vi "app - Scott Thing.vi"() -> ()   [LabVIEW 2014]
uses:
  <vilib>/event_ctls.llb/eventvkey.ctl
  freq file -- file select control.ctl
  freq file -- file select folder control.ctl
  cursor winow.ctl
  fit function selector control.ctl
  countdown control.ctl
  cursor window action.ctl
  array transformation action.ctl
  container action.ctl
  cursor action.ctl
  save-read action.ctl
  generate linear region.vi
  tale of three indices.vi
  Q -- check range -- i -- real.vi
  linear interpolation iiii- complex.vi
  Q -- check range -- i -- integer.vi
  file -- 9w path.vi
  file -- open-create folder.vi
  command stack.vi
  tale of three indices -- check state.vi
  Q - not nan -- real.vi
  Q - not nan -- integer.vi
  <vilib>/regexp/Match Regular Expression.xnode
panel:
  in  "plot fit?":bool
  out "slope temp vs time (K/min)":dbl=-0.40469687981224706
  out "slope vs temp (1/K)":dbl=-8.892288495374525e-05
  out "slope vs time (1/min)":dbl=3.599048348461236e-05
  in  "phase":dbl=10.0
  out "phase of Frequency vs Temperature phase(rad)":dbl=10.0
  out "phase of Frequency (rad)":dbl=10.0
  out "phase of Temperature (rad)":dbl=10.0
  in  "window/period":dbl=114.59
  out "averaging window (min)":dbl=114.59
  in  "cursor bracket: delta freq vs time":T1={"left"=45.0, "right "=55.0, "center"=50.0, "window"=10.0, "cursors"=[1, 2, 3], "relative"=0, "absolute"=0, "fixed vertical offset"=0.0, "vertical offset"=0.0, "skew"=0.0, "default window frac"=0.1, "kind"=enum."skewed", "skew.left"=0.5, "skew.right"=0.5, "Plot ref"=refnum, "wing order"=enum."forw"}
  in  "period (min)":dbl(slide) scale=0.0..200.0
  in  "Lockin wave: Period (min)":dbl=114.59
  in  "Lockin wave: Amplitude":dbl=10.0
  in  "Lockin wave: Phase":dbl=1.0
  in  "lockin (l)":bool
  out "Plot: lockin":cluster{dbl[], dbl[]}[](graph)
  in  "Numeric sort  folder names ?":bool=TRUE
  in  "Tab : other":enum32{"indicators", "other"}(tab)
  in  "file 2 (red)":T2={"from file "="890_mo", "load"=TRUE, "read from file list"=3, "folder kind"=enum."monitor"} {"read from file list" items=["363_mo", "524_mo", "997_mo", "1331_mo", "2102_mo", "2312_mo", "3182_mo", "3227_mo", "3271_mo", "3302_mo", "3420_mo", "3606_mo", "3780_mo", "3988_mo"]}
  in  "file 1 (blue)":T2={"from file "="890_mo", "load"=TRUE, "read from file list"=3, "folder kind"=enum."monitor"} {"read from file list" items=["363_mo", "524_mo", "997_mo", "1331_mo", "2102_mo", "2312_mo", "3182_mo", "3227_mo", "3271_mo", "3302_mo", "3420_mo", "3606_mo", "3780_mo", "3988_mo"]}
  out "time (min)":dbl=513.2382892057026
  in  "open (o)":bool
  in  "plot (p)":bool
  in  "plot type":T4(ring)=enum."plot vs Temperature"
  out "temperature (K)":dbl=369.642
  out "frequency (kHz)":dbl
  in  "sweep folder 2":u16(ring)=1 items=["0_test", "1_cooling", "2_heating", "3_heating"]
  in  "sweep folder 1":u16(ring)=1 items=["0_test", "1_cooling", "2_heating", "3_heating"]
  out "folder --OK":bool=TRUE
  out "file 2 -- OK":bool=TRUE
  out "file 1 -- OK":bool=TRUE
  out "best fit parameters":dbl[](array[numeric])=[61.921916709262796, 419.38173960994607, 184.61021915940464]
  in  "fit dataset":enum16{"fit blue dataset", "fit red  dataset"}(ring)
  in  "fit using":T5=enum."einstein"
  out "current index":dbl=1431.5698546544484
  out "Char":i16=122
  out "VKey":T6
  in  "Tab: timer":enum32{"timer ON", "timer OFF"}(tab)=enum."timer OFF"
  in  "timer  \"update\"":dbl(slide) min=-543877211.0 max=2129711151.0 step=0.010000000000000002 scale=0.0..100.0 scale format="%#3_3f"
  in  "Tab : all":enum32{"everything", "everything else"}(tab)
  out "Plot: gamma vs time":cluster{dbl[], dbl[]}[](graph)=[{[0.0, 0.8321000039577484, 1.8338100016117096, 2.665260002017021, 3.6651000007987022, 4.500330001115799, 5.331799998879433, 6.33356000483036, 7.165059998631477, 8.166830003261566, 9.000310003757477, 9.665630005300045, 10.330900005996227, 10.99813000112772, 11.66363000124693, 12.332860000431538, 12.833530001342297, 13.498850002884865, 14.16593000292778, 14.831310003995895, 15.49855000525713, 16.165710002183914, 16.833000004291534, 17.33186000585556, 17.999030001461506, 18.66473000496626, 19.331909999251366, 19.99728000164032, 20.66636000573635, 21.33170000463724, 21.83238000422716, 22.49956000596285, 23.164850004017353, 23.83196000009775, 24.499110005795956, 25.16636000573635, 25.831660002470016, 26.332430005073547, 26.999680005013943, 27.664980001747608, 28.334049999713898, 28.99931000173092, 29.66651000082493, 30.331810005009174, 30.832600004971027, 31.49796000123024, 32.165130004286766, 32.83415000140667, 33.49946000427008, 34.166660003364086, 34.831980004906654, 35.332830004394054, 35.99830999970436, 36.667510002851486, 37.33306000381708, 38.000459998846054, 38.665800005197525, 39.33306000381708, 39.83373000472784, 40.499180004000664, 41.16650000214577, 41.83186000585556, 42.500900000333786, 43.166230000555515, 43.833429999649525, 44.332249999046326, 44.99943000078201, 45.66485000401735, 46.334100000560284, 46.99949999898672, 47.6666100025177, 47.982130005955696, 48.19973000138998, 48.33212999999523, 48.83280999958515, 49.50008000433445, 50.16723000258207, 50.834449999034405, 51.49991000443697, 52.16526000201702, 52.83435000479221, 53.33311000466347, 54.0003300011158, 54.66745000332594, 55.33465000241995, 55.999960005283356, 56.66730999946594, 57.33255000412464, 57.83314999938011, 58.50026000291109, 59.16743000596762, 59.83455999940634, 60.499880000948906, 61.16710000485182, 61.83251000195742, 62.33313000202179, 63.002580001950264, 63.667830005288124, 64.33306000381708, 65.00022999942303, 65.66740000247955, 66.33458000421524, 66.83331000059843, 67.50053000450134, 68.16818000376225, 68.83345000445843, 69.50058000534773, 70.16781000047922, 70.83495999872684, 71.33570000529289, 72.00148000568151, 72.66678000241518, 73.33390000462532, 74.00111000239849, 74.66830000281334, 75.33545999974012, 75.8344499990344, 76.50161000341177, 77.16766000539064, 77.83305000513792, 78.50201000273228, 79.1691600009799, 79.83455000072718, 80.33545999974012, 81.00163000077009, 81.66701000183821, 82.33430000394583, 83.00148000568151, 83.66863000392914, 84.33410999923944, 84.8347800001502, 85.50213000178337, 86.1676000058651, 86.83668000251055, 87.5020300000906, 88.16926000267267, 88.83460000157356, 89.33528000116348, 90.00060000270605, 90.66975000500679, 91.33512999862432, 92.00230000168085, 92.66781000047922, 93.33495999872684, 93.83557999879122, 94.50090999901295, 95.16995999962091, 95.83531000465155, 96.50246000289917, 97.16770000010729, 97.83486000448465, 98.33560000360012, 99.00268000364304, 99.66976000368595, 100.33528000116348, 101.06157000362873], [0.67588, 0.61324, 0.61184, 0.55194, 0.46793, 0.65413, 0.45513, 0.53529, 0.55031, 0.6231, 0.46874, 0.37253, 0.62303, 0.69213, 0.48939, 0.40586, 0.51301, 0.53019, 0.56055, 0.71323, 0.4387, 0.62201, 0.52499, 0.55885, 0.40767, 0.52913, 0.37684, 0.81007, 0.55143, 0.62952, 0.6183, 0.66198, 0.55623, 0.41442, 0.51737, 0.49906, 0.34582, 0.55383, 0.50878, 0.61849, 0.46781, 0.4094, 0.56226, 0.53343, 0.56808, 0.59375, 0.55552, 0.52806, 0.55238, 0.57542, 0.55055, 0.51811, 0.56627, 0.47603, 0.60558, 0.5391, 0.53997, 0.46766, 0.50061, 0.55367, 0.54193, 0.57806, 0.59611, 0.41969, 0.60712, 0.57486, 0.54068, 0.49673, 0.41822, 0.51666, 0.53002, 0.54071, 0.54381, 0.50371, 0.47659, 0.55271, 0.51695, 0.5054, 0.48403, 0.63454, 0.46381, 0.54415, 0.49407, 0.50294, 0.59277, 0.51141, 0.49779, 0.62513, 0.58238, 0.60458, 0.51762, 0.49132, 0.62927, 0.59156, 0.61264, 0.58665, 0.49186, 0.57277, 0.60236, 0.52088, 0.54777, 0.34446, 0.60604, 0.56549, 0.5463, 0.62015, 0.55365, 0.55892, 0.59896, 0.5722, 0.6325, 0.52149, 0.60349, 0.49569, 0.5793, 0.6434, 0.58917, 0.56576, 0.62655, 0.66023, 0.6492, 0.64793, 0.66476, 0.61207, 0.69632, 0.68932, 0.6121, 0.67902, 0.6855, 0.6683, 0.68361, 0.71016, 0.731, 0.74257, 0.71351, 0.66404, 0.77828, 0.66741, 0.65821, 0.79074, 0.71129, 0.70388, 0.704, 0.73193, 0.7246, 0.75975, 0.76321, 0.75811, 0.69136, 0.71185, 0.76071, 0.59918, 0.80205, 0.73634, 0.77823, 0.66937]}]
  out "Plot: temp vs time":cluster{dbl[], dbl[]}[](graph)=[{[0.0, 0.8321000039577484, 1.8338100016117096, 2.665260002017021, 3.6651000007987022, 4.500330001115799, 5.331799998879433, 6.33356000483036, 7.165059998631477, 8.166830003261566, 9.000310003757477, 9.665630005300045, 10.330900005996227, 10.99813000112772, 11.66363000124693, 12.332860000431538, 12.833530001342297, 13.498850002884865, 14.16593000292778, 14.831310003995895, 15.49855000525713, 16.165710002183914, 16.833000004291534, 17.33186000585556, 17.999030001461506, 18.66473000496626, 19.331909999251366, 19.99728000164032, 20.66636000573635, 21.33170000463724, 21.83238000422716, 22.49956000596285, 23.164850004017353, 23.83196000009775, 24.499110005795956, 25.16636000573635, 25.831660002470016, 26.332430005073547, 26.999680005013943, 27.664980001747608, 28.334049999713898, 28.99931000173092, 29.66651000082493, 30.331810005009174, 30.832600004971027, 31.49796000123024, 32.165130004286766, 32.83415000140667, 33.49946000427008, 34.166660003364086, 34.831980004906654, 35.332830004394054, 35.99830999970436, 36.667510002851486, 37.33306000381708, 38.000459998846054, 38.665800005197525, 39.33306000381708, 39.83373000472784, 40.499180004000664, 41.16650000214577, 41.83186000585556, 42.500900000333786, 43.166230000555515, 43.833429999649525, 44.332249999046326, 44.99943000078201, 45.66485000401735, 46.334100000560284, 46.99949999898672, 47.6666100025177, 47.982130005955696, 48.19973000138998, 48.33212999999523, 48.83280999958515, 49.50008000433445, 50.16723000258207, 50.834449999034405, 51.49991000443697, 52.16526000201702, 52.83435000479221, 53.33311000466347, 54.0003300011158, 54.66745000332594, 55.33465000241995, 55.999960005283356, 56.66730999946594, 57.33255000412464, 57.83314999938011, 58.50026000291109, 59.16743000596762, 59.83455999940634, 60.499880000948906, 61.16710000485182, 61.83251000195742, 62.33313000202179, 63.002580001950264, 63.667830005288124, 64.33306000381708, 65.00022999942303, 65.66740000247955, 66.33458000421524, 66.83331000059843, 67.50053000450134, 68.16818000376225, 68.83345000445843, 69.50058000534773, 70.16781000047922, 70.83495999872684, 71.33570000529289, 72.00148000568151, 72.66678000241518, 73.33390000462532, 74.00111000239849, 74.66830000281334, 75.33545999974012, 75.8344499990344, 76.50161000341177, 77.16766000539064, 77.83305000513792, 78.50201000273228, 79.1691600009799, 79.83455000072718, 80.33545999974012, 81.00163000077009, 81.66701000183821, 82.33430000394583, 83.00148000568151, 83.66863000392914, 84.33410999923944, 84.8347800001502, 85.50213000178337, 86.1676000058651, 86.83668000251055, 87.5020300000906, 88.16926000267267, 88.83460000157356, 89.33528000116348, 90.00060000270605, 90.66975000500679, 91.33512999862432, 92.00230000168085, 92.66781000047922, 93.33495999872684, 93.83557999879122, 94.50090999901295, 95.16995999962091, 95.83531000465155, 96.50246000289917, 97.16770000010729, 97.83486000448465, 98.33560000360012, 99.00268000364304, 99.66976000368595, 100.33528000116348, 101.06157000362873], [306.859, 306.865, 306.758, 306.535, 306.258, 305.982, 305.68, 305.339, 305.019, 304.645, 304.3, 303.965, 303.725, 303.462, 303.2, 302.977, 302.732, 302.46, 302.218, 301.952, 301.736, 301.437, 301.186, 300.927, 300.684, 300.432, 300.14, 299.908, 299.659, 299.377, 299.116, 298.866, 298.605, 298.361, 298.06, 297.801, 297.575, 297.284, 297.046, 296.769, 296.514, 296.224, 295.989, 295.704, 295.444, 295.182, 294.904, 294.655, 294.379, 294.131, 293.821, 293.569, 293.289, 293.052, 292.75, 292.472, 292.244, 291.771, 291.552, 291.447, 291.24, 290.887, 290.534, 290.294, 290.021, 289.766, 289.473, 289.178, 288.91, 288.631, 288.354, 288.354, 288.354, 288.104, 287.889, 287.626, 287.379, 287.122, 286.875, 286.621, 286.387, 286.134, 285.896, 285.647, 285.385, 285.15, 284.882, 284.657, 284.389, 284.134, 283.88, 283.628, 283.367, 283.103, 282.849, 282.604, 282.322, 282.068, 281.815, 281.535, 281.296, 281.007, 280.774, 280.511, 280.222, 279.971, 279.687, 279.464, 279.175, 278.934, 278.648, 278.394, 278.136, 277.881, 277.611, 277.368, 277.093, 276.842, 276.498, 276.243, 276.006, 275.757, 275.403, 275.18, 274.898, 274.596, 274.32, 274.065, 273.786, 273.463, 273.219, 272.879, 272.671, 272.345, 272.085, 271.771, 271.544, 271.227, 270.941, 270.676, 270.353, 270.079, 269.753, 269.519, 269.228, 268.904, 268.594, 268.306, 268.058, 267.801, 267.52, 267.286, 267.028, 266.779, 266.494, 266.257]}]
  out "Plot: gamma":cluster{dbl[], dbl[]}[](graph)=[{[306.859, 306.865, 306.758, 306.535, 306.258, 305.982, 305.68, 305.339, 305.019, 304.645, 304.3, 303.965, 303.725, 303.462, 303.2, 302.977, 302.732, 302.46, 302.218, 301.952, 301.736, 301.437, 301.186, 300.927, 300.684, 300.432, 300.14, 299.908, 299.659, 299.377, 299.116, 298.866, 298.605, 298.361, 298.06, 297.801, 297.575, 297.284, 297.046, 296.769, 296.514, 296.224, 295.989, 295.704, 295.444, 295.182, 294.904, 294.655, 294.379, 294.131, 293.821, 293.569, 293.289, 293.052, 292.75, 292.472, 292.244, 291.771, 291.552, 291.447, 291.24, 290.887, 290.534, 290.294, 290.021, 289.766, 289.473, 289.178, 288.91, 288.631, 288.354, 288.354, 288.354, 288.104, 287.889, 287.626, 287.379, 287.122, 286.875, 286.621, 286.387, 286.134, 285.896, 285.647, 285.385, 285.15, 284.882, 284.657, 284.389, 284.134, 283.88, 283.628, 283.367, 283.103, 282.849, 282.604, 282.322, 282.068, 281.815, 281.535, 281.296, 281.007, 280.774, 280.511, 280.222, 279.971, 279.687, 279.464, 279.175, 278.934, 278.648, 278.394, 278.136, 277.881, 277.611, 277.368, 277.093, 276.842, 276.498, 276.243, 276.006, 275.757, 275.403, 275.18, 274.898, 274.596, 274.32, 274.065, 273.786, 273.463, 273.219, 272.879, 272.671, 272.345, 272.085, 271.771, 271.544, 271.227, 270.941, 270.676, 270.353, 270.079, 269.753, 269.519, 269.228, 268.904, 268.594, 268.306, 268.058, 267.801, 267.52, 267.286, 267.028, 266.779, 266.494, 266.257], [0.67588, 0.61324, 0.61184, 0.55194, 0.46793, 0.65413, 0.45513, 0.53529, 0.55031, 0.6231, 0.46874, 0.37253, 0.62303, 0.69213, 0.48939, 0.40586, 0.51301, 0.53019, 0.56055, 0.71323, 0.4387, 0.62201, 0.52499, 0.55885, 0.40767, 0.52913, 0.37684, 0.81007, 0.55143, 0.62952, 0.6183, 0.66198, 0.55623, 0.41442, 0.51737, 0.49906, 0.34582, 0.55383, 0.50878, 0.61849, 0.46781, 0.4094, 0.56226, 0.53343, 0.56808, 0.59375, 0.55552, 0.52806, 0.55238, 0.57542, 0.55055, 0.51811, 0.56627, 0.47603, 0.60558, 0.5391, 0.53997, 0.46766, 0.50061, 0.55367, 0.54193, 0.57806, 0.59611, 0.41969, 0.60712, 0.57486, 0.54068, 0.49673, 0.41822, 0.51666, 0.53002, 0.54071, 0.54381, 0.50371, 0.47659, 0.55271, 0.51695, 0.5054, 0.48403, 0.63454, 0.46381, 0.54415, 0.49407, 0.50294, 0.59277, 0.51141, 0.49779, 0.62513, 0.58238, 0.60458, 0.51762, 0.49132, 0.62927, 0.59156, 0.61264, 0.58665, 0.49186, 0.57277, 0.60236, 0.52088, 0.54777, 0.34446, 0.60604, 0.56549, 0.5463, 0.62015, 0.55365, 0.55892, 0.59896, 0.5722, 0.6325, 0.52149, 0.60349, 0.49569, 0.5793, 0.6434, 0.58917, 0.56576, 0.62655, 0.66023, 0.6492, 0.64793, 0.66476, 0.61207, 0.69632, 0.68932, 0.6121, 0.67902, 0.6855, 0.6683, 0.68361, 0.71016, 0.731, 0.74257, 0.71351, 0.66404, 0.77828, 0.66741, 0.65821, 0.79074, 0.71129, 0.70388, 0.704, 0.73193, 0.7246, 0.75975, 0.76321, 0.75811, 0.69136, 0.71185, 0.76071, 0.59918, 0.80205, 0.73634, 0.77823, 0.66937]}, {[306.859, 306.865, 306.758, 306.535, 306.258, 305.982, 305.68, 305.339, 305.019, 304.645, 304.3, 303.965, 303.725, 303.462, 303.2, 302.977, 302.732, 302.46, 302.218, 301.952, 301.736, 301.437, 301.186, 300.927, 300.684, 300.432, 300.14, 299.908, 299.659, 299.377, 299.116, 298.866, 298.605, 298.361, 298.06, 297.801, 297.575, 297.284, 297.046, 296.769, 296.514, 296.224, 295.989, 295.704, 295.444, 295.182, 294.904, 294.655, 294.379, 294.131, 293.821, 293.569, 293.289, 293.052, 292.75, 292.472, 292.244, 291.771, 291.552, 291.447, 291.24, 290.887, 290.534, 290.294, 290.021, 289.766, 289.473, 289.178, 288.91, 288.631, 288.354, 288.354, 288.354, 288.104, 287.889, 287.626, 287.379, 287.122, 286.875, 286.621, 286.387, 286.134, 285.896, 285.647, 285.385, 285.15, 284.882, 284.657, 284.389, 284.134, 283.88, 283.628, 283.367, 283.103, 282.849, 282.604, 282.322, 282.068, 281.815, 281.535, 281.296, 281.007, 280.774, 280.511, 280.222, 279.971, 279.687, 279.464, 279.175, 278.934, 278.648, 278.394, 278.136, 277.881, 277.611, 277.368, 277.093, 276.842, 276.498, 276.243, 276.006, 275.757, 275.403, 275.18, 274.898, 274.596, 274.32, 274.065, 273.786, 273.463, 273.219, 272.879, 272.671, 272.345, 272.085, 271.771, 271.544, 271.227, 270.941, 270.676, 270.353, 270.079, 269.753, 269.519, 269.228, 268.904, 268.594, 268.306, 268.058, 267.801, 267.52, 267.286, 267.028, 266.779, 266.494, 266.257], [0.67588, 0.61324, 0.61184, 0.55194, 0.46793, 0.65413, 0.45513, 0.53529, 0.55031, 0.6231, 0.46874, 0.37253, 0.62303, 0.69213, 0.48939, 0.40586, 0.51301, 0.53019, 0.56055, 0.71323, 0.4387, 0.62201, 0.52499, 0.55885, 0.40767, 0.52913, 0.37684, 0.81007, 0.55143, 0.62952, 0.6183, 0.66198, 0.55623, 0.41442, 0.51737, 0.49906, 0.34582, 0.55383, 0.50878, 0.61849, 0.46781, 0.4094, 0.56226, 0.53343, 0.56808, 0.59375, 0.55552, 0.52806, 0.55238, 0.57542, 0.55055, 0.51811, 0.56627, 0.47603, 0.60558, 0.5391, 0.53997, 0.46766, 0.50061, 0.55367, 0.54193, 0.57806, 0.59611, 0.41969, 0.60712, 0.57486, 0.54068, 0.49673, 0.41822, 0.51666, 0.53002, 0.54071, 0.54381, 0.50371, 0.47659, 0.55271, 0.51695, 0.5054, 0.48403, 0.63454, 0.46381, 0.54415, 0.49407, 0.50294, 0.59277, 0.51141, 0.49779, 0.62513, 0.58238, 0.60458, 0.51762, 0.49132, 0.62927, 0.59156, 0.61264, 0.58665, 0.49186, 0.57277, 0.60236, 0.52088, 0.54777, 0.34446, 0.60604, 0.56549, 0.5463, 0.62015, 0.55365, 0.55892, 0.59896, 0.5722, 0.6325, 0.52149, 0.60349, 0.49569, 0.5793, 0.6434, 0.58917, 0.56576, 0.62655, 0.66023, 0.6492, 0.64793, 0.66476, 0.61207, 0.69632, 0.68932, 0.6121, 0.67902, 0.6855, 0.6683, 0.68361, 0.71016, 0.731, 0.74257, 0.71351, 0.66404, 0.77828, 0.66741, 0.65821, 0.79074, 0.71129, 0.70388, 0.704, 0.73193, 0.7246, 0.75975, 0.76321, 0.75811, 0.69136, 0.71185, 0.76071, 0.59918, 0.80205, 0.73634, 0.77823, 0.66937]}]
  out "Plot: freq vs time":cluster{dbl[], dbl[]}[](graph)=[{[0.0, 0.8321000039577484, 1.8338100016117096, 2.665260002017021, 3.6651000007987022, 4.500330001115799, 5.331799998879433, 6.33356000483036, 7.165059998631477, 8.166830003261566, 9.000310003757477, 9.665630005300045, 10.330900005996227, 10.99813000112772, 11.66363000124693, 12.332860000431538, 12.833530001342297, 13.498850002884865, 14.16593000292778, 14.831310003995895, 15.49855000525713, 16.165710002183914, 16.833000004291534, 17.33186000585556, 17.999030001461506, 18.66473000496626, 19.331909999251366, 19.99728000164032, 20.66636000573635, 21.33170000463724, 21.83238000422716, 22.49956000596285, 23.164850004017353, 23.83196000009775, 24.499110005795956, 25.16636000573635, 25.831660002470016, 26.332430005073547, 26.999680005013943, 27.664980001747608, 28.334049999713898, 28.99931000173092, 29.66651000082493, 30.331810005009174, 30.832600004971027, 31.49796000123024, 32.165130004286766, 32.83415000140667, 33.49946000427008, 34.166660003364086, 34.831980004906654, 35.332830004394054, 35.99830999970436, 36.667510002851486, 37.33306000381708, 38.000459998846054, 38.665800005197525, 39.33306000381708, 39.83373000472784, 40.499180004000664, 41.16650000214577, 41.83186000585556, 42.500900000333786, 43.166230000555515, 43.833429999649525, 44.332249999046326, 44.99943000078201, 45.66485000401735, 46.334100000560284, 46.99949999898672, 47.6666100025177, 47.982130005955696, 48.19973000138998, 48.33212999999523, 48.83280999958515, 49.50008000433445, 50.16723000258207, 50.834449999034405, 51.49991000443697, 52.16526000201702, 52.83435000479221, 53.33311000466347, 54.0003300011158, 54.66745000332594, 55.33465000241995, 55.999960005283356, 56.66730999946594, 57.33255000412464, 57.83314999938011, 58.50026000291109, 59.16743000596762, 59.83455999940634, 60.499880000948906, 61.16710000485182, 61.83251000195742, 62.33313000202179, 63.002580001950264, 63.667830005288124, 64.33306000381708, 65.00022999942303, 65.66740000247955, 66.33458000421524, 66.83331000059843, 67.50053000450134, 68.16818000376225, 68.83345000445843, 69.50058000534773, 70.16781000047922, 70.83495999872684, 71.33570000529289, 72.00148000568151, 72.66678000241518, 73.33390000462532, 74.00111000239849, 74.66830000281334, 75.33545999974012, 75.8344499990344, 76.50161000341177, 77.16766000539064, 77.83305000513792, 78.50201000273228, 79.1691600009799, 79.83455000072718, 80.33545999974012, 81.00163000077009, 81.66701000183821, 82.33430000394583, 83.00148000568151, 83.66863000392914, 84.33410999923944, 84.8347800001502, 85.50213000178337, 86.1676000058651, 86.83668000251055, 87.5020300000906, 88.16926000267267, 88.83460000157356, 89.33528000116348, 90.00060000270605, 90.66975000500679, 91.33512999862432, 92.00230000168085, 92.66781000047922, 93.33495999872684, 93.83557999879122, 94.50090999901295, 95.16995999962091, 95.83531000465155, 96.50246000289917, 97.16770000010729, 97.83486000448465, 98.33560000360012, 99.00268000364304, 99.66976000368595, 100.33528000116348, 101.06157000362873], [889.69584, 889.68006, 889.69255, 889.71739, 889.74198, 889.76413, 889.80509, 889.81267, 889.81316, 889.83768, 889.86543, 889.88159, 889.92939, 889.90105, 889.9266, 889.95895, 889.97981, 889.97629, 889.98977, 890.00084, 890.03646, 890.03085, 890.07055, 890.08625, 890.08815, 890.10584, 890.1305, 890.12034, 890.16981, 890.17806, 890.23087, 890.20536, 890.20895, 890.26922, 890.27026, 890.2972, 890.29936, 890.33499, 890.34497, 890.35023, 890.38545, 890.40235, 890.4306, 890.43746, 890.47621, 890.46739, 890.48511, 890.50908, 890.54654, 890.5436, 890.5795, 890.5927, 890.60709, 890.62748, 890.63996, 890.66299, 890.6957, 890.71803, 890.72686, 890.73173, 890.77668, 890.76873, 890.81256, 890.82914, 890.85272, 890.85398, 890.87546, 890.9031, 890.91221, 890.94167, 890.96276, 890.9639, 890.96372, 890.98604, 891.01233, 891.02469, 891.04793, 891.07006, 891.08048, 891.09899, 891.12512, 891.12536, 891.15654, 891.16879, 891.18905, 891.19959, 891.22995, 891.24753, 891.26162, 891.28335, 891.28567, 891.31231, 891.32899, 891.34942, 891.36424, 891.3683, 891.38547, 891.40448, 891.44656, 891.44488, 891.47205, 891.20744, 891.49222, 891.54408, 891.54113, 891.572, 891.58143, 891.60752, 891.60686, 891.64483, 891.65678, 891.68328, 891.6931, 891.70715, 891.72898, 891.75723, 891.77658, 891.78596, 891.81354, 891.83601, 891.85493, 891.86836, 891.88286, 891.89968, 891.93208, 891.95223, 891.96891, 891.99329, 892.01204, 892.02476, 892.05135, 892.06661, 892.06875, 892.09013, 892.12382, 892.14219, 892.1629, 892.18968, 892.20319, 892.24544, 892.25704, 892.28489, 892.29651, 892.31599, 892.33983, 892.34947, 892.37436, 892.40785, 892.42946, 892.4521, 892.46919, 892.48367, 892.49371, 892.51877, 892.53774, 892.56817]}]
  out "Plot: frequency":cluster{dbl[], dbl[]}[](graph)=[{[306.859, 306.865, 306.758, 306.535, 306.258, 305.982, 305.68, 305.339, 305.019, 304.645, 304.3, 303.965, 303.725, 303.462, 303.2, 302.977, 302.732, 302.46, 302.218, 301.952, 301.736, 301.437, 301.186, 300.927, 300.684, 300.432, 300.14, 299.908, 299.659, 299.377, 299.116, 298.866, 298.605, 298.361, 298.06, 297.801, 297.575, 297.284, 297.046, 296.769, 296.514, 296.224, 295.989, 295.704, 295.444, 295.182, 294.904, 294.655, 294.379, 294.131, 293.821, 293.569, 293.289, 293.052, 292.75, 292.472, 292.244, 291.771, 291.552, 291.447, 291.24, 290.887, 290.534, 290.294, 290.021, 289.766, 289.473, 289.178, 288.91, 288.631, 288.354, 288.354, 288.354, 288.104, 287.889, 287.626, 287.379, 287.122, 286.875, 286.621, 286.387, 286.134, 285.896, 285.647, 285.385, 285.15, 284.882, 284.657, 284.389, 284.134, 283.88, 283.628, 283.367, 283.103, 282.849, 282.604, 282.322, 282.068, 281.815, 281.535, 281.296, 281.007, 280.774, 280.511, 280.222, 279.971, 279.687, 279.464, 279.175, 278.934, 278.648, 278.394, 278.136, 277.881, 277.611, 277.368, 277.093, 276.842, 276.498, 276.243, 276.006, 275.757, 275.403, 275.18, 274.898, 274.596, 274.32, 274.065, 273.786, 273.463, 273.219, 272.879, 272.671, 272.345, 272.085, 271.771, 271.544, 271.227, 270.941, 270.676, 270.353, 270.079, 269.753, 269.519, 269.228, 268.904, 268.594, 268.306, 268.058, 267.801, 267.52, 267.286, 267.028, 266.779, 266.494, 266.257], [889.69584, 889.68006, 889.69255, 889.71739, 889.74198, 889.76413, 889.80509, 889.81267, 889.81316, 889.83768, 889.86543, 889.88159, 889.92939, 889.90105, 889.9266, 889.95895, 889.97981, 889.97629, 889.98977, 890.00084, 890.03646, 890.03085, 890.07055, 890.08625, 890.08815, 890.10584, 890.1305, 890.12034, 890.16981, 890.17806, 890.23087, 890.20536, 890.20895, 890.26922, 890.27026, 890.2972, 890.29936, 890.33499, 890.34497, 890.35023, 890.38545, 890.40235, 890.4306, 890.43746, 890.47621, 890.46739, 890.48511, 890.50908, 890.54654, 890.5436, 890.5795, 890.5927, 890.60709, 890.62748, 890.63996, 890.66299, 890.6957, 890.71803, 890.72686, 890.73173, 890.77668, 890.76873, 890.81256, 890.82914, 890.85272, 890.85398, 890.87546, 890.9031, 890.91221, 890.94167, 890.96276, 890.9639, 890.96372, 890.98604, 891.01233, 891.02469, 891.04793, 891.07006, 891.08048, 891.09899, 891.12512, 891.12536, 891.15654, 891.16879, 891.18905, 891.19959, 891.22995, 891.24753, 891.26162, 891.28335, 891.28567, 891.31231, 891.32899, 891.34942, 891.36424, 891.3683, 891.38547, 891.40448, 891.44656, 891.44488, 891.47205, 891.20744, 891.49222, 891.54408, 891.54113, 891.572, 891.58143, 891.60752, 891.60686, 891.64483, 891.65678, 891.68328, 891.6931, 891.70715, 891.72898, 891.75723, 891.77658, 891.78596, 891.81354, 891.83601, 891.85493, 891.86836, 891.88286, 891.89968, 891.93208, 891.95223, 891.96891, 891.99329, 892.01204, 892.02476, 892.05135, 892.06661, 892.06875, 892.09013, 892.12382, 892.14219, 892.1629, 892.18968, 892.20319, 892.24544, 892.25704, 892.28489, 892.29651, 892.31599, 892.33983, 892.34947, 892.37436, 892.40785, 892.42946, 892.4521, 892.46919, 892.48367, 892.49371, 892.51877, 892.53774, 892.56817]}, {[306.859, 306.865, 306.758, 306.535, 306.258, 305.982, 305.68, 305.339, 305.019, 304.645, 304.3, 303.965, 303.725, 303.462, 303.2, 302.977, 302.732, 302.46, 302.218, 301.952, 301.736, 301.437, 301.186, 300.927, 300.684, 300.432, 300.14, 299.908, 299.659, 299.377, 299.116, 298.866, 298.605, 298.361, 298.06, 297.801, 297.575, 297.284, 297.046, 296.769, 296.514, 296.224, 295.989, 295.704, 295.444, 295.182, 294.904, 294.655, 294.379, 294.131, 293.821, 293.569, 293.289, 293.052, 292.75, 292.472, 292.244, 291.771, 291.552, 291.447, 291.24, 290.887, 290.534, 290.294, 290.021, 289.766, 289.473, 289.178, 288.91, 288.631, 288.354, 288.354, 288.354, 288.104, 287.889, 287.626, 287.379, 287.122, 286.875, 286.621, 286.387, 286.134, 285.896, 285.647, 285.385, 285.15, 284.882, 284.657, 284.389, 284.134, 283.88, 283.628, 283.367, 283.103, 282.849, 282.604, 282.322, 282.068, 281.815, 281.535, 281.296, 281.007, 280.774, 280.511, 280.222, 279.971, 279.687, 279.464, 279.175, 278.934, 278.648, 278.394, 278.136, 277.881, 277.611, 277.368, 277.093, 276.842, 276.498, 276.243, 276.006, 275.757, 275.403, 275.18, 274.898, 274.596, 274.32, 274.065, 273.786, 273.463, 273.219, 272.879, 272.671, 272.345, 272.085, 271.771, 271.544, 271.227, 270.941, 270.676, 270.353, 270.079, 269.753, 269.519, 269.228, 268.904, 268.594, 268.306, 268.058, 267.801, 267.52, 267.286, 267.028, 266.779, 266.494, 266.257], [889.69584, 889.68006, 889.69255, 889.71739, 889.74198, 889.76413, 889.80509, 889.81267, 889.81316, 889.83768, 889.86543, 889.88159, 889.92939, 889.90105, 889.9266, 889.95895, 889.97981, 889.97629, 889.98977, 890.00084, 890.03646, 890.03085, 890.07055, 890.08625, 890.08815, 890.10584, 890.1305, 890.12034, 890.16981, 890.17806, 890.23087, 890.20536, 890.20895, 890.26922, 890.27026, 890.2972, 890.29936, 890.33499, 890.34497, 890.35023, 890.38545, 890.40235, 890.4306, 890.43746, 890.47621, 890.46739, 890.48511, 890.50908, 890.54654, 890.5436, 890.5795, 890.5927, 890.60709, 890.62748, 890.63996, 890.66299, 890.6957, 890.71803, 890.72686, 890.73173, 890.77668, 890.76873, 890.81256, 890.82914, 890.85272, 890.85398, 890.87546, 890.9031, 890.91221, 890.94167, 890.96276, 890.9639, 890.96372, 890.98604, 891.01233, 891.02469, 891.04793, 891.07006, 891.08048, 891.09899, 891.12512, 891.12536, 891.15654, 891.16879, 891.18905, 891.19959, 891.22995, 891.24753, 891.26162, 891.28335, 891.28567, 891.31231, 891.32899, 891.34942, 891.36424, 891.3683, 891.38547, 891.40448, 891.44656, 891.44488, 891.47205, 891.20744, 891.49222, 891.54408, 891.54113, 891.572, 891.58143, 891.60752, 891.60686, 891.64483, 891.65678, 891.68328, 891.6931, 891.70715, 891.72898, 891.75723, 891.77658, 891.78596, 891.81354, 891.83601, 891.85493, 891.86836, 891.88286, 891.89968, 891.93208, 891.95223, 891.96891, 891.99329, 892.01204, 892.02476, 892.05135, 892.06661, 892.06875, 892.09013, 892.12382, 892.14219, 892.1629, 892.18968, 892.20319, 892.24544, 892.25704, 892.28489, 892.29651, 892.31599, 892.33983, 892.34947, 892.37436, 892.40785, 892.42946, 892.4521, 892.46919, 892.48367, 892.49371, 892.51877, 892.53774, 892.56817]}, {[306.859, 306.865, 306.758, 306.535, 306.258, 305.982, 305.68, 305.339, 305.019, 304.645, 304.3, 303.965, 303.725, 303.462, 303.2, 302.977, 302.732, 302.46, 302.218, 301.952, 301.736, 301.437, 301.186, 300.927, 300.684, 300.432, 300.14, 299.908, 299.659, 299.377, 299.116, 298.866, 298.605, 298.361, 298.06, 297.801, 297.575, 297.284, 297.046, 296.769, 296.514, 296.224, 295.989, 295.704, 295.444, 295.182, 294.904, 294.655, 294.379, 294.131, 293.821, 293.569, 293.289, 293.052, 292.75, 292.472, 292.244, 291.771, 291.552, 291.447, 291.24, 290.887, 290.534, 290.294, 290.021, 289.766, 289.473, 289.178, 288.91, 288.631, 288.354, 288.354, 288.354, 288.104, 287.889, 287.626, 287.379, 287.122, 286.875, 286.621, 286.387, 286.134, 285.896, 285.647, 285.385, 285.15, 284.882, 284.657, 284.389, 284.134, 283.88, 283.628, 283.367, 283.103, 282.849, 282.604, 282.322, 282.068, 281.815, 281.535, 281.296, 281.007, 280.774, 280.511, 280.222, 279.971, 279.687, 279.464, 279.175, 278.934, 278.648, 278.394, 278.136, 277.881, 277.611, 277.368, 277.093, 276.842, 276.498, 276.243, 276.006, 275.757, 275.403, 275.18, 274.898, 274.596, 274.32, 274.065, 273.786, 273.463, 273.219, 272.879, 272.671, 272.345, 272.085, 271.771, 271.544, 271.227, 270.941, 270.676, 270.353, 270.079, 269.753, 269.519, 269.228, 268.904, 268.594, 268.306, 268.058, 267.801, 267.52, 267.286, 267.028, 266.779, 266.494, 266.257], [570.2268269908692, 570.2400535112981, 570.0041828919524, 569.5126179393131, 568.9020492485238, 568.293717838797, 567.6281177621656, 566.876610474574, 566.171429915419, 565.3473070426576, 564.587141311005, 563.8490596480553, 563.3203152743283, 562.7409289284184, 562.1637761789564, 561.6725596037392, 561.1329078353073, 560.5338157540311, 560.0008279496419, 559.4150122842709, 558.9393358485567, 558.2809111876567, 557.7282181275183, 557.1579393994253, 556.6229180617343, 556.0681096330096, 555.4252727779038, 554.9145536178556, 554.3664386572701, 553.7457165304331, 553.171251200151, 552.6210267025464, 552.0466233598377, 551.5096620032419, 550.8473013177035, 550.2773970629929, 549.7801318596763, 549.1398833614178, 548.6162734429868, 548.006895693501, 547.4459483952983, 546.8080459681299, 546.291154491278, 545.664321581304, 545.0925080223979, 544.5163288085155, 543.9049992980612, 543.3574733145706, 542.7506121888769, 542.2053482848695, 541.5238105844371, 540.9698210157459, 540.3543135724759, 539.8333606049329, 539.169570362039, 538.5585715114518, 538.0574931299626, 537.0180576955482, 536.5368346856114, 536.3061198313321, 535.851298153545, 535.0757340020174, 534.300232607959, 533.7730154878564, 533.1733414952065, 532.613240646205, 531.9697146847699, 531.321840361095, 530.7333016604363, 530.1206457254603, 529.5124212635792, 529.5124212635792, 529.5124212635792, 528.9635162504065, 528.4914838279942, 527.9141000571886, 527.3718750762423, 526.8077314613829, 526.2655715221489, 525.708080097659, 525.1945156563919, 524.6392840115748, 524.1170021138493, 523.5706132562343, 522.9957336250801, 522.4801284084958, 521.8921550370692, 521.3985503585072, 520.8106477876426, 520.2512987495651, 519.6941781032982, 519.1414787112122, 518.5690763531383, 517.9901323319139, 517.4331538681354, 516.8959442695048, 516.2776457779006, 515.7207760293832, 515.166134017826, 514.552342186182, 514.0284613708559, 513.3950244395973, 512.8843634820904, 512.3079886115614, 511.67467838184996, 511.12467883289094, 510.502411368327, 510.01383186237047, 509.3806922392472, 508.8527470088059, 508.226265695658, 507.66991934199706, 507.10484943632076, 506.54638765251946, 505.95511596666734, 505.4230074186946, 504.8208681793691, 504.27131757679274, 503.51820818618506, 502.95998853984645, 502.44120676686646, 501.89619307927956, 501.12141717804076, 500.63339011921533, 500.0162859635069, 499.3554679298154, 498.75158903238935, 498.19369789341613, 497.5833439890978, 496.8767919878564, 496.3430916184932, 495.599470817134, 495.1445844202257, 494.43169042383516, 493.86317113561313, 493.176629920022, 492.6803464114658, 491.98735160177364, 491.3621792468444, 490.78295637786283, 490.0770192071422, 489.47822564970915, 488.7658535979936, 488.25456015341325, 487.618768928462, 486.9109405410003, 486.23375955274724, 485.6046912754734, 485.06303594470444, 484.50176523690385, 483.8881285866703, 483.3771673951809, 482.81384083052166, 482.2702059815308, 481.64802263700415, 481.1306682656006]}]
  out "Plot: delta frequency":T7(graph)=[{"Temperature (K) Array"=[306.859, 306.865, 306.758, 306.535, 306.258, 305.982, 305.68, 305.339, 305.019, 304.645, 304.3, 303.965, 303.725, 303.462, 303.2, 302.977, 302.732, 302.46, 302.218, 301.952, 301.736, 301.437, 301.186, 300.927, 300.684, 300.432, 300.14, 299.908, 299.659, 299.377, 299.116, 298.866, 298.605, 298.361, 298.06, 297.801, 297.575, 297.284, 297.046, 296.769, 296.514, 296.224, 295.989, 295.704, 295.444, 295.182, 294.904, 294.655, 294.379, 294.131, 293.821, 293.569, 293.289, 293.052, 292.75, 292.472, 292.244, 291.771, 291.552, 291.447, 291.24, 290.887, 290.534, 290.294, 290.021, 289.766, 289.473, 289.178, 288.91, 288.631, 288.354, 288.354, 288.354, 288.104, 287.889, 287.626, 287.379, 287.122, 286.875, 286.621, 286.387, 286.134, 285.896, 285.647, 285.385, 285.15, 284.882, 284.657, 284.389, 284.134, 283.88, 283.628, 283.367, 283.103, 282.849, 282.604, 282.322, 282.068, 281.815, 281.535, 281.296, 281.007, 280.774, 280.511, 280.222, 279.971, 279.687, 279.464, 279.175, 278.934, 278.648, 278.394, 278.136, 277.881, 277.611, 277.368, 277.093, 276.842, 276.498, 276.243, 276.006, 275.757, 275.403, 275.18, 274.898, 274.596, 274.32, 274.065, 273.786, 273.463, 273.219, 272.879, 272.671, 272.345, 272.085, 271.771, 271.544, 271.227, 270.941, 270.676, 270.353, 270.079, 269.753, 269.519, 269.228, 268.904, 268.594, 268.306, 268.058, 267.801, 267.52, 267.286, 267.028, 266.779, 266.494, 266.257], "freq out"=[319.4690130091308, 319.4400064887019, 319.6883671080476, 320.2047720606869, 320.83993075147623, 321.47041216120306, 322.1769722378343, 322.936059525426, 323.641730084581, 324.4903729573424, 325.27828868899496, 326.0325303519446, 326.6090747256717, 327.16012107158167, 327.76282382104364, 328.2863903962608, 328.8469021646928, 329.4424742459688, 329.9889420503581, 330.5858277157291, 331.0971241514434, 331.7499388123433, 332.34233187248174, 332.9283106005746, 333.4652319382658, 334.03773036699033, 334.70522722209614, 335.2057863821444, 335.80337134272986, 336.43234346956683, 337.059618799849, 337.58433329745367, 338.1623266401623, 338.7595579967581, 339.42295868229655, 340.01980293700706, 340.51922814032366, 341.19510663858216, 341.7286965570132, 342.34333430649906, 342.9395016047017, 343.59430403187, 344.139445508722, 344.773138418696, 345.3837019776022, 345.95106119148454, 346.5801107019388, 347.15160668542944, 347.7959278111232, 348.33825171513047, 349.05568941556294, 349.62287898425416, 350.25277642752405, 350.7941193950671, 351.4703896379609, 352.1044184885483, 352.6382068700374, 353.69997230445176, 354.19002531438855, 354.42561016866784, 354.925381846455, 355.6929959979826, 356.512327392041, 357.0561245121437, 357.6793785047935, 358.240739353795, 358.9057453152301, 359.58125963890495, 360.1789083395637, 360.8210242745397, 361.4503387364208, 361.45147873642077, 361.45129873642077, 362.02252374959346, 362.5208461720058, 363.1105899428113, 363.67605492375765, 364.2623285386171, 364.8149084778511, 365.3909099023409, 365.93060434360814, 366.4860759884252, 367.0395378861507, 367.59817674376563, 368.19331637491985, 368.7194615915041, 369.33779496293084, 369.84897964149275, 370.45097221235744, 371.03205125043496, 371.59149189670177, 372.1708312887878, 372.7599136468617, 373.35928766808615, 373.9310861318646, 374.4723557304952, 375.10782422209945, 375.6837039706169, 376.28042598217394, 376.89253781381797, 377.4435886291441, 377.81241556040277, 378.60785651790957, 379.2360913884386, 379.86645161815, 380.44732116710907, 381.07901863167297, 381.59368813762956, 382.2261677607528, 382.79208299119404, 383.430514304342, 384.0133606580029, 384.5882505636792, 385.1607623474805, 385.77386403333264, 386.3342225813054, 386.9557118206309, 387.5146424232073, 388.2953318138149, 388.87602146015354, 389.4137232331335, 389.9721669207205, 390.7614428219593, 391.26628988078465, 391.91579403649314, 392.5967620701846, 393.2173209676107, 393.7995921065839, 394.4286960109022, 395.1479680121436, 395.70825838150677, 396.467139182866, 396.9241655797743, 397.6584395761649, 398.2606488643869, 398.96556007997805, 399.48255358853424, 400.2023283982263, 400.84101075315556, 401.4624836221372, 402.18002079285776, 402.8066643502909, 403.5306564020064, 404.0614298465868, 404.72106107153803, 405.4385294589997, 406.1406004472528, 406.80315872452667, 407.3664240552955, 407.9503347630961, 408.58106141332973, 409.10650260481907, 409.6798691694783, 410.2485640184692, 410.88971736299584, 411.4375017343994]}, {"Temperature (K) Array"=[306.859, 306.865, 306.758, 306.535, 306.258, 305.982, 305.68, 305.339, 305.019, 304.645, 304.3, 303.965, 303.725, 303.462, 303.2, 302.977, 302.732, 302.46, 302.218, 301.952, 301.736, 301.437, 301.186, 300.927, 300.684, 300.432, 300.14, 299.908, 299.659, 299.377, 299.116, 298.866, 298.605, 298.361, 298.06, 297.801, 297.575, 297.284, 297.046, 296.769, 296.514, 296.224, 295.989, 295.704, 295.444, 295.182, 294.904, 294.655, 294.379, 294.131, 293.821, 293.569, 293.289, 293.052, 292.75, 292.472, 292.244, 291.771, 291.552, 291.447, 291.24, 290.887, 290.534, 290.294, 290.021, 289.766, 289.473, 289.178, 288.91, 288.631, 288.354, 288.354, 288.354, 288.104, 287.889, 287.626, 287.379, 287.122, 286.875, 286.621, 286.387, 286.134, 285.896, 285.647, 285.385, 285.15, 284.882, 284.657, 284.389, 284.134, 283.88, 283.628, 283.367, 283.103, 282.849, 282.604, 282.322, 282.068, 281.815, 281.535, 281.296, 281.007, 280.774, 280.511, 280.222, 279.971, 279.687, 279.464, 279.175, 278.934, 278.648, 278.394, 278.136, 277.881, 277.611, 277.368, 277.093, 276.842, 276.498, 276.243, 276.006, 275.757, 275.403, 275.18, 274.898, 274.596, 274.32, 274.065, 273.786, 273.463, 273.219, 272.879, 272.671, 272.345, 272.085, 271.771, 271.544, 271.227, 270.941, 270.676, 270.353, 270.079, 269.753, 269.519, 269.228, 268.904, 268.594, 268.306, 268.058, 267.801, 267.52, 267.286, 267.028, 266.779, 266.494, 266.257], "freq out"=[319.4690130091308, 319.4400064887019, 319.6883671080476, 320.2047720606869, 320.83993075147623, 321.47041216120306, 322.1769722378343, 322.936059525426, 323.641730084581, 324.4903729573424, 325.27828868899496, 326.0325303519446, 326.6090747256717, 327.16012107158167, 327.76282382104364, 328.2863903962608, 328.8469021646928, 329.4424742459688, 329.9889420503581, 330.5858277157291, 331.0971241514434, 331.7499388123433, 332.34233187248174, 332.9283106005746, 333.4652319382658, 334.03773036699033, 334.70522722209614, 335.2057863821444, 335.80337134272986, 336.43234346956683, 337.059618799849, 337.58433329745367, 338.1623266401623, 338.7595579967581, 339.42295868229655, 340.01980293700706, 340.51922814032366, 341.19510663858216, 341.7286965570132, 342.34333430649906, 342.9395016047017, 343.59430403187, 344.139445508722, 344.773138418696, 345.3837019776022, 345.95106119148454, 346.5801107019388, 347.15160668542944, 347.7959278111232, 348.33825171513047, 349.05568941556294, 349.62287898425416, 350.25277642752405, 350.7941193950671, 351.4703896379609, 352.1044184885483, 352.6382068700374, 353.69997230445176, 354.19002531438855, 354.42561016866784, 354.925381846455, 355.6929959979826, 356.512327392041, 357.0561245121437, 357.6793785047935, 358.240739353795, 358.9057453152301, 359.58125963890495, 360.1789083395637, 360.8210242745397, 361.4503387364208, 361.45147873642077, 361.45129873642077, 362.02252374959346, 362.5208461720058, 363.1105899428113, 363.67605492375765, 364.2623285386171, 364.8149084778511, 365.3909099023409, 365.93060434360814, 366.4860759884252, 367.0395378861507, 367.59817674376563, 368.19331637491985, 368.7194615915041, 369.33779496293084, 369.84897964149275, 370.45097221235744, 371.03205125043496, 371.59149189670177, 372.1708312887878, 372.7599136468617, 373.35928766808615, 373.9310861318646, 374.4723557304952, 375.10782422209945, 375.6837039706169, 376.28042598217394, 376.89253781381797, 377.4435886291441, 377.81241556040277, 378.60785651790957, 379.2360913884386, 379.86645161815, 380.44732116710907, 381.07901863167297, 381.59368813762956, 382.2261677607528, 382.79208299119404, 383.430514304342, 384.0133606580029, 384.5882505636792, 385.1607623474805, 385.77386403333264, 386.3342225813054, 386.9557118206309, 387.5146424232073, 388.2953318138149, 388.87602146015354, 389.4137232331335, 389.9721669207205, 390.7614428219593, 391.26628988078465, 391.91579403649314, 392.5967620701846, 393.2173209676107, 393.7995921065839, 394.4286960109022, 395.1479680121436, 395.70825838150677, 396.467139182866, 396.9241655797743, 397.6584395761649, 398.2606488643869, 398.96556007997805, 399.48255358853424, 400.2023283982263, 400.84101075315556, 401.4624836221372, 402.18002079285776, 402.8066643502909, 403.5306564020064, 404.0614298465868, 404.72106107153803, 405.4385294589997, 406.1406004472528, 406.80315872452667, 407.3664240552955, 407.9503347630961, 408.58106141332973, 409.10650260481907, 409.6798691694783, 410.2485640184692, 410.88971736299584, 411.4375017343994]}]
  out "Plot: delta freq vs time":cluster{dbl[], dbl[]}[](graph)=[{[0.0, 0.8321000039577484, 1.8338100016117096, 2.665260002017021, 3.6651000007987022, 4.500330001115799, 5.331799998879433, 6.33356000483036, 7.165059998631477, 8.166830003261566, 9.000310003757477, 9.665630005300045, 10.330900005996227, 10.99813000112772, 11.66363000124693, 12.332860000431538, 12.833530001342297, 13.498850002884865, 14.16593000292778, 14.831310003995895, 15.49855000525713, 16.165710002183914, 16.833000004291534, 17.33186000585556, 17.999030001461506, 18.66473000496626, 19.331909999251366, 19.99728000164032, 20.66636000573635, 21.33170000463724, 21.83238000422716, 22.49956000596285, 23.164850004017353, 23.83196000009775, 24.499110005795956, 25.16636000573635, 25.831660002470016, 26.332430005073547, 26.999680005013943, 27.664980001747608, 28.334049999713898, 28.99931000173092, 29.66651000082493, 30.331810005009174, 30.832600004971027, 31.49796000123024, 32.165130004286766, 32.83415000140667, 33.49946000427008, 34.166660003364086, 34.831980004906654, 35.332830004394054, 35.99830999970436, 36.667510002851486, 37.33306000381708, 38.000459998846054, 38.665800005197525, 39.33306000381708, 39.83373000472784, 40.499180004000664, 41.16650000214577, 41.83186000585556, 42.500900000333786, 43.166230000555515, 43.833429999649525, 44.332249999046326, 44.99943000078201, 45.66485000401735, 46.334100000560284, 46.99949999898672, 47.6666100025177, 47.982130005955696, 48.19973000138998, 48.33212999999523, 48.83280999958515, 49.50008000433445, 50.16723000258207, 50.834449999034405, 51.49991000443697, 52.16526000201702, 52.83435000479221, 53.33311000466347, 54.0003300011158, 54.66745000332594, 55.33465000241995, 55.999960005283356, 56.66730999946594, 57.33255000412464, 57.83314999938011, 58.50026000291109, 59.16743000596762, 59.83455999940634, 60.499880000948906, 61.16710000485182, 61.83251000195742, 62.33313000202179, 63.002580001950264, 63.667830005288124, 64.33306000381708, 65.00022999942303, 65.66740000247955, 66.33458000421524, 66.83331000059843, 67.50053000450134, 68.16818000376225, 68.83345000445843, 69.50058000534773, 70.16781000047922, 70.83495999872684, 71.33570000529289, 72.00148000568151, 72.66678000241518, 73.33390000462532, 74.00111000239849, 74.66830000281334, 75.33545999974012, 75.8344499990344, 76.50161000341177, 77.16766000539064, 77.83305000513792, 78.50201000273228, 79.1691600009799, 79.83455000072718, 80.33545999974012, 81.00163000077009, 81.66701000183821, 82.33430000394583, 83.00148000568151, 83.66863000392914, 84.33410999923944, 84.8347800001502, 85.50213000178337, 86.1676000058651, 86.83668000251055, 87.5020300000906, 88.16926000267267, 88.83460000157356, 89.33528000116348, 90.00060000270605, 90.66975000500679, 91.33512999862432, 92.00230000168085, 92.66781000047922, 93.33495999872684, 93.83557999879122, 94.50090999901295, 95.16995999962091, 95.83531000465155, 96.50246000289917, 97.16770000010729, 97.83486000448465, 98.33560000360012, 99.00268000364304, 99.66976000368595, 100.33528000116348, 101.06157000362873], [319.4690130091308, 319.4400064887019, 319.6883671080476, 320.2047720606869, 320.83993075147623, 321.47041216120306, 322.1769722378343, 322.936059525426, 323.641730084581, 324.4903729573424, 325.27828868899496, 326.0325303519446, 326.6090747256717, 327.16012107158167, 327.76282382104364, 328.2863903962608, 328.8469021646928, 329.4424742459688, 329.9889420503581, 330.5858277157291, 331.0971241514434, 331.7499388123433, 332.34233187248174, 332.9283106005746, 333.4652319382658, 334.03773036699033, 334.70522722209614, 335.2057863821444, 335.80337134272986, 336.43234346956683, 337.059618799849, 337.58433329745367, 338.1623266401623, 338.7595579967581, 339.42295868229655, 340.01980293700706, 340.51922814032366, 341.19510663858216, 341.7286965570132, 342.34333430649906, 342.9395016047017, 343.59430403187, 344.139445508722, 344.773138418696, 345.3837019776022, 345.95106119148454, 346.5801107019388, 347.15160668542944, 347.7959278111232, 348.33825171513047, 349.05568941556294, 349.62287898425416, 350.25277642752405, 350.7941193950671, 351.4703896379609, 352.1044184885483, 352.6382068700374, 353.69997230445176, 354.19002531438855, 354.42561016866784, 354.925381846455, 355.6929959979826, 356.512327392041, 357.0561245121437, 357.6793785047935, 358.240739353795, 358.9057453152301, 359.58125963890495, 360.1789083395637, 360.8210242745397, 361.4503387364208, 361.45147873642077, 361.45129873642077, 362.02252374959346, 362.5208461720058, 363.1105899428113, 363.67605492375765, 364.2623285386171, 364.8149084778511, 365.3909099023409, 365.93060434360814, 366.4860759884252, 367.0395378861507, 367.59817674376563, 368.19331637491985, 368.7194615915041, 369.33779496293084, 369.84897964149275, 370.45097221235744, 371.03205125043496, 371.59149189670177, 372.1708312887878, 372.7599136468617, 373.35928766808615, 373.9310861318646, 374.4723557304952, 375.10782422209945, 375.6837039706169, 376.28042598217394, 376.89253781381797, 377.4435886291441, 377.81241556040277, 378.60785651790957, 379.2360913884386, 379.86645161815, 380.44732116710907, 381.07901863167297, 381.59368813762956, 382.2261677607528, 382.79208299119404, 383.430514304342, 384.0133606580029, 384.5882505636792, 385.1607623474805, 385.77386403333264, 386.3342225813054, 386.9557118206309, 387.5146424232073, 388.2953318138149, 388.87602146015354, 389.4137232331335, 389.9721669207205, 390.7614428219593, 391.26628988078465, 391.91579403649314, 392.5967620701846, 393.2173209676107, 393.7995921065839, 394.4286960109022, 395.1479680121436, 395.70825838150677, 396.467139182866, 396.9241655797743, 397.6584395761649, 398.2606488643869, 398.96556007997805, 399.48255358853424, 400.2023283982263, 400.84101075315556, 401.4624836221372, 402.18002079285776, 402.8066643502909, 403.5306564020064, 404.0614298465868, 404.72106107153803, 405.4385294589997, 406.1406004472528, 406.80315872452667, 407.3664240552955, 407.9503347630961, 408.58106141332973, 409.10650260481907, 409.6798691694783, 410.2485640184692, 410.88971736299584, 411.4375017343994]}]
  in  "main folder":path=path "D:/Technique/RUS/URuSi/DU45-325"
  in  "file 2 path":path=path "D:/Technique/RUS/URuSi/DU45-325/1_cooling/9w/monitor/890_mo.dat"
  in  "file 1 path":path=path "D:/Technique/RUS/URuSi/DU45-325/1_cooling/9w/monitor/890_mo.dat"
  in  "folder 2":path=path "D:/Technique/RUS/URuSi/DU45-325/1_cooling"
  in  "folder 1":path=path "D:/Technique/RUS/URuSi/DU45-325/1_cooling"
  in  "cursor bracket: freq":T1={"left"=287.88733, "right "=291.64867000000004, "center"=289.76800000000003, "window"=3.7613400000000072, "cursors"=[1, 2, 3], "relative"=0, "absolute"=0, "fixed vertical offset"=0.0, "vertical offset"=0.0, "skew"=0.0, "default window frac"=0.1, "kind"=enum."symmetric", "skew.left"=0.5, "skew.right"=0.5, "Plot ref"=refnum, "wing order"=enum."forw"}
  in  "cursor bracket: temp vs time":T1={"left"=45.0, "right "=55.0, "center"=50.0, "window"=10.0, "cursors"=[1, 2, 3], "relative"=0, "absolute"=0, "fixed vertical offset"=0.0, "vertical offset"=0.0, "skew"=0.0, "default window frac"=0.1, "kind"=enum."skewed", "skew.left"=0.5, "skew.right"=0.5, "Plot ref"=refnum, "wing order"=enum."forw"}
  out "delta freq (file 1) (kHz)":dbl[](array[numeric])=[319.4690130091308, 319.4400064887019, 319.6883671080476, 320.2047720606869, 320.83993075147623, 321.47041216120306, 322.1769722378343, 322.936059525426, 323.641730084581, 324.4903729573424, 325.27828868899496, 326.0325303519446, 326.6090747256717, 327.16012107158167, 327.76282382104364, 328.2863903962608, 328.8469021646928, 329.4424742459688, 329.9889420503581, 330.5858277157291, 331.0971241514434, 331.7499388123433, 332.34233187248174, 332.9283106005746, 333.4652319382658, 334.03773036699033, 334.70522722209614, 335.2057863821444, 335.80337134272986, 336.43234346956683, 337.059618799849, 337.58433329745367, 338.1623266401623, 338.7595579967581, 339.42295868229655, 340.01980293700706, 340.51922814032366, 341.19510663858216, 341.7286965570132, 342.34333430649906, 342.9395016047017, 343.59430403187, 344.139445508722, 344.773138418696, 345.3837019776022, 345.95106119148454, 346.5801107019388, 347.15160668542944, 347.7959278111232, 348.33825171513047, 349.05568941556294, 349.62287898425416, 350.25277642752405, 350.7941193950671, 351.4703896379609, 352.1044184885483, 352.6382068700374, 353.69997230445176, 354.19002531438855, 354.42561016866784, 354.925381846455, 355.6929959979826, 356.512327392041, 357.0561245121437, 357.6793785047935, 358.240739353795, 358.9057453152301, 359.58125963890495, 360.1789083395637, 360.8210242745397, 361.4503387364208, 361.45147873642077, 361.45129873642077, 362.02252374959346, 362.5208461720058, 363.1105899428113, 363.67605492375765, 364.2623285386171, 364.8149084778511, 365.3909099023409, 365.93060434360814, 366.4860759884252, 367.0395378861507, 367.59817674376563, 368.19331637491985, 368.7194615915041, 369.33779496293084, 369.84897964149275, 370.45097221235744, 371.03205125043496, 371.59149189670177, 372.1708312887878, 372.7599136468617, 373.35928766808615, 373.9310861318646, 374.4723557304952, 375.10782422209945, 375.6837039706169, 376.28042598217394, 376.89253781381797, 377.4435886291441, 377.81241556040277, 378.60785651790957, 379.2360913884386, 379.86645161815, 380.44732116710907, 381.07901863167297, 381.59368813762956, 382.2261677607528, 382.79208299119404, 383.430514304342, 384.0133606580029, 384.5882505636792, 385.1607623474805, 385.77386403333264, 386.3342225813054, 386.9557118206309, 387.5146424232073, 388.2953318138149, 388.87602146015354, 389.4137232331335, 389.9721669207205, 390.7614428219593, 391.26628988078465, 391.91579403649314, 392.5967620701846, 393.2173209676107, 393.7995921065839, 394.4286960109022, 395.1479680121436, 395.70825838150677, 396.467139182866, 396.9241655797743, 397.6584395761649, 398.2606488643869, 398.96556007997805, 399.48255358853424, 400.2023283982263, 400.84101075315556, 401.4624836221372, 402.18002079285776, 402.8066643502909, 403.5306564020064, 404.0614298465868, 404.72106107153803, 405.4385294589997, 406.1406004472528, 406.80315872452667, 407.3664240552955, 407.9503347630961, 408.58106141332973, 409.10650260481907, 409.6798691694783, 410.2485640184692, 410.88971736299584, 411.4375017343994]
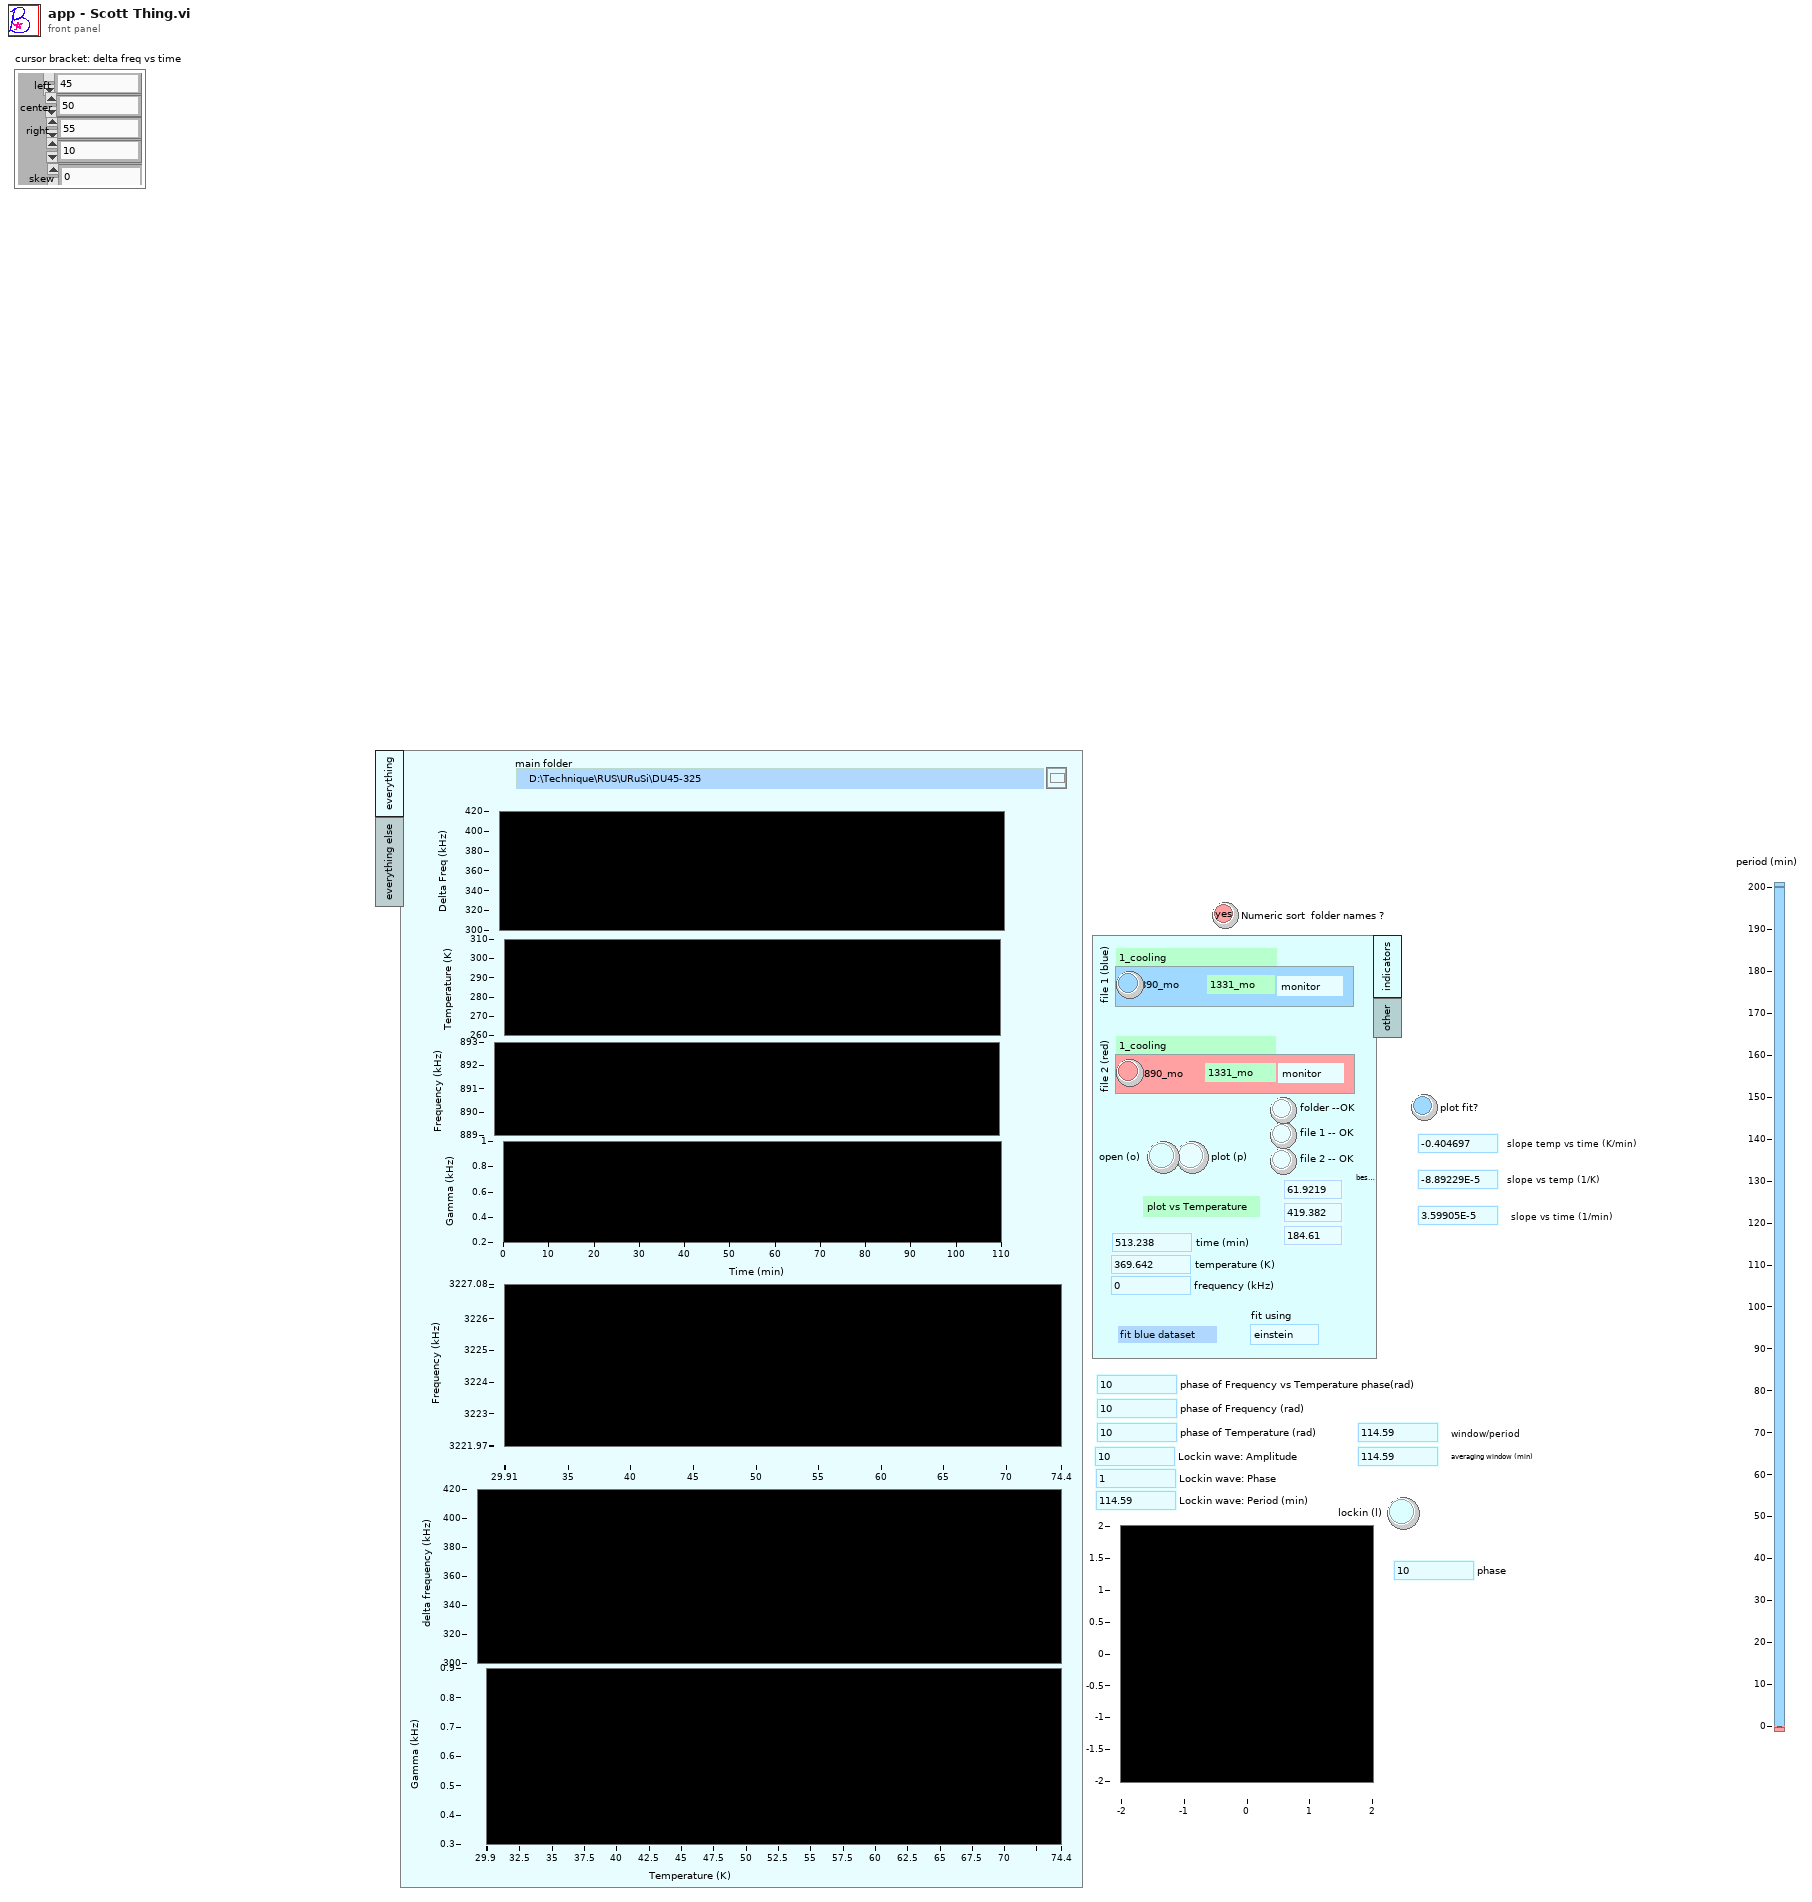
[diagram p1: front panel]
types:
  T1 = typedef "cursor winow.ctl" = cluster{"left":dbl, "right ":dbl, "center":dbl, "window":dbl, "cursors":i32[], "relative":i32, "absolute":i32, "fixed vertical offset":dbl, "vertical offset":dbl, "skew":dbl, "default window frac":dbl, "kind":enum16{"symmetric", "skewed", "fancy"}, "skew.left":dbl, "skew.right":dbl, "Plot ref":refnum<vi>, "wing order":enum16{"forw", "back"}}
  T2 = typedef "freq file -- file select control.ctl" = cluster{"from file ":string, "load":bool, "read from file list":u16, "folder kind":T3}
  T3 = typedef "freq file -- file select folder control.ctl" = enum16{"monitor", "9w"}
  T4 = enum16{"plot vs Magnetic Field", "plot vs Temperature"}
  T5 = typedef "fit function selector control.ctl" = enum16{"linear", "varshni", "varshni5", "LogMinusT", "hyperbola", "einstein", "sine", "sine2theta", "cos2theta"}
  T6 = typedef "eventvkey.ctl" = enum16{"ASCII", "Enter", "Return", "Shift", "Ctrl", "Alt", "Cmd", "Opt", "Caps", "NumLock", "Clear", "Break", "Up", "Down", "Left", "Right", "Insert", "Delete", "Home", "End", "PageUp", "PageDown", "Escape", "Help", "Pause", "ScrollLock", "F1", "F2", "F3", "F4", "F5", "F6", "F7", "F8", "F9", "F10", "F11", "F12", "F13", "F14", "F15", "F16", "F17", "F18", "F19", "F20", "F21", "F22", "F23", "F24", "Play", "VolumeUp", "VolumeDown", "Mute", "Two Byte Char"}
  T7 = cluster{"Temperature (K) Array":dbl[], "freq out":dbl[]}[]
  T8 = typedef "cursor window action.ctl" = enum16{"balance", "h. offset change", "cursor moves", "change center", "change window", "init", "check", "reset", "set y to middle", "idle", "-write all Y", "-write left.X", "-write center.X", "-write right.X", "-write all X", "-change center", "-change window", "-change skew", "-read cursor 2", "-read cursor 1", "-read cursor 0", "-read all cursors", "-reset", "-read plot scale", "-set y to middle", "-Q: center.Y is visible", "-Q: window is visible", "-parse center.Y", "-right left from center", "-left move", "-right move", "-set center.Y", "-empty", "-set cursors to default", "-check", "-write center.Y", "-copy cursor 1", "-copy cursor 0", "-copy cursor 2", "move right", "move left", "shrink", "broaden", "skew up", "skew down", "-write plot scale", "zoom X", "change cen&win", "zoom to all data"}
  T9 = typedef "countdown control.ctl" = enum16{"check", "start", "reset cont", "stop", "reset once"}
  T10 = typedef "container action.ctl" = enum16{"get", "read file", "plot", "init", "set"}
  T11 = typedef "array transformation action.ctl" = enum16{"remove mean", "nomalize (by abs magn)", "rotate phase"}
  T12 = cluster{"time (min) array":dbl[], "Temperature (K) Array":dbl[]}
  T13 = cluster{"time (min) array":dbl[], "Frequency (kHz) Array":dbl[]}
  T14 = cluster{"time (min) array":dbl[], "Gamma (kHz) Array":dbl[]}
  T15 = cluster{"time (min) array":dbl[], "Temperature (K) Array":dbl[]}[]
  T16 = cluster{"time (min) array":dbl[], "Frequency (kHz) Array":dbl[]}[]
  T17 = cluster{"time (min) array":dbl[], "Gamma (kHz) Array":dbl[]}[]
  T18 = typedef "cursor action.ctl" = enum16{"range", "read", "write", "check", "zoom out", "smart zoom out"}
  T19 = cluster{"Temperature (K) Array":dbl[], "Gamma (kHz) Array":dbl[]}
  T20 = cluster{"Temperature (K) Array":dbl[], "Frequency (kHz) Array":dbl[]}
  T21 = cluster{"Temperature (K) Array":dbl[], "Frequency (kHz) Array":dbl[]}[]
  T22 = cluster{"Temperature (K) Array":dbl[], "Gamma (kHz) Array":dbl[]}[]
  T23 = cluster{"Temperature (K) Array":dbl[], "freq out":dbl[]}
  T24 = cluster{"Field (T) Array":dbl[], "Gamma (kHz) Array":dbl[]}
  T25 = cluster{"Field (T) Array":dbl[], "Frequency (kHz) Array":dbl[]}
  T26 = cluster{"Field (T) Array":dbl[], "Frequency (kHz) Array":dbl[]}[]
  T27 = cluster{"Field (T) Array":dbl[], "Gamma (kHz) Array":dbl[]}[]
  T28 = typedef "save-read action.ctl" = enum16{"update save list", "update read list", "init", "check", "lookup read number", "lookup write number", "copy read from read ring", "saved file dirty", "saved file clean", "read file OK", "read file not OK", "nearest right", "nearest left", "increment read from", "copy read to save", "init save file", "erase event", "save event", "read event", "set save file", "decrement read from"}
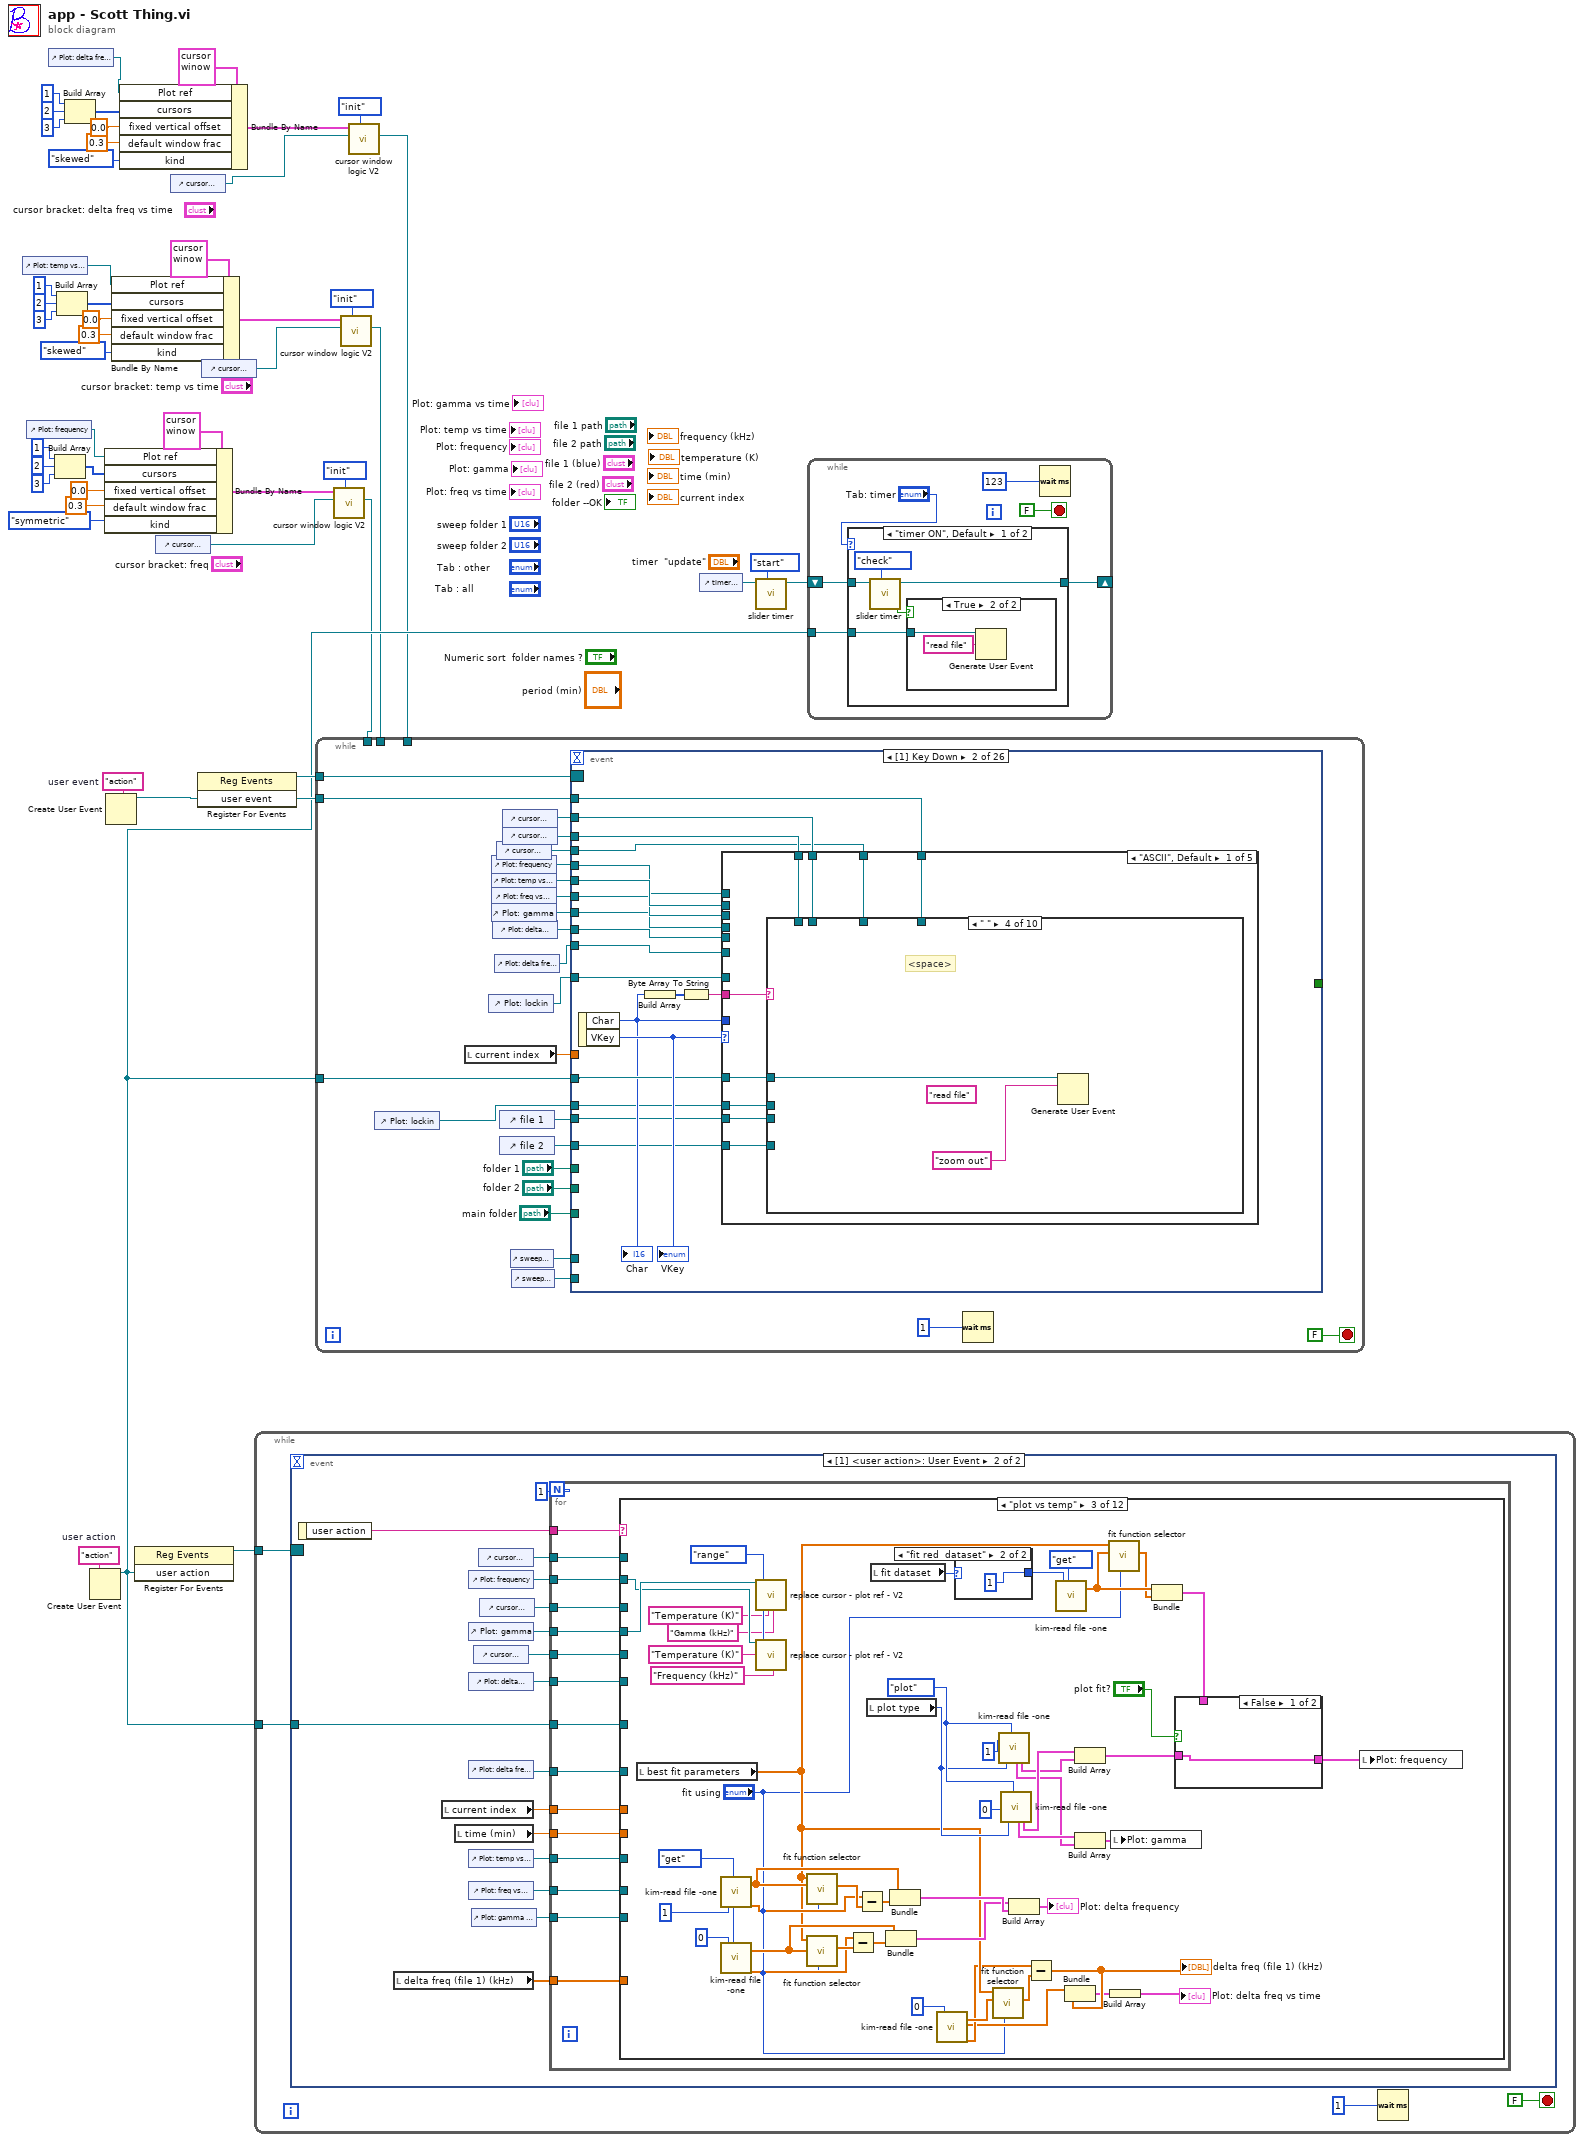
[diagram p0: block diagram]
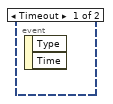
[diagram p4: hidden frame]
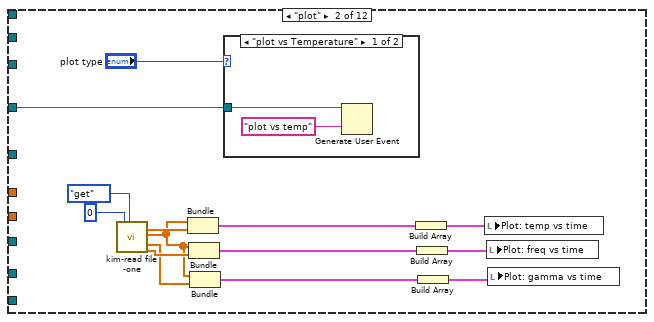
[diagram p6: hidden frame]
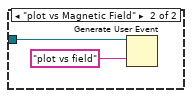
[diagram p7: hidden frame]
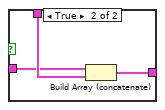
[diagram p8: hidden frame]
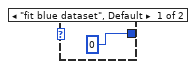
[diagram p9: hidden frame]
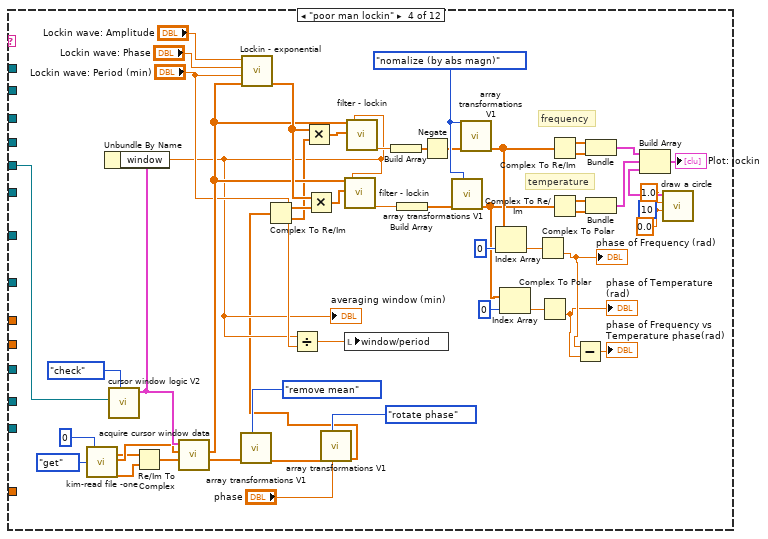
[diagram p10: hidden frame]
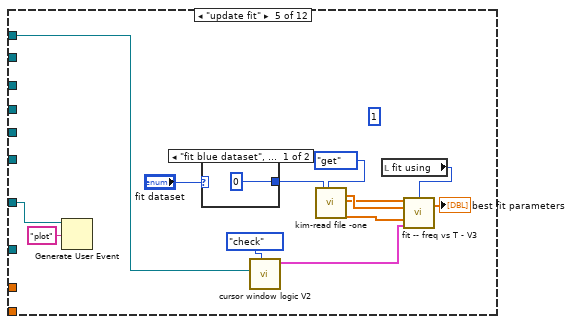
[diagram p11: hidden frame]
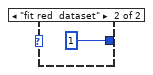
[diagram p12: hidden frame]
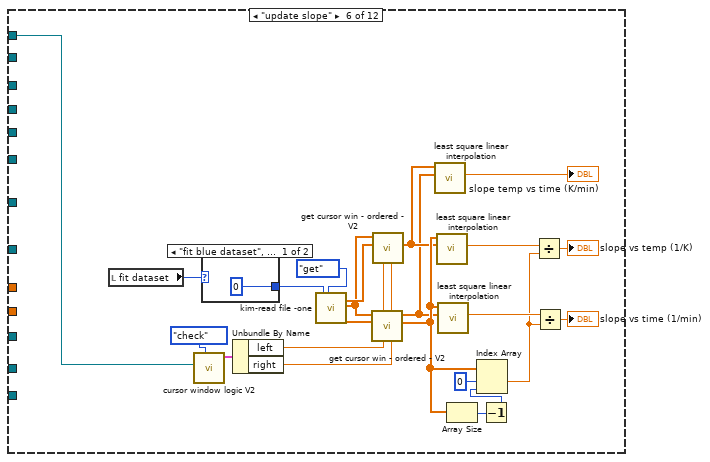
[diagram p13: hidden frame]
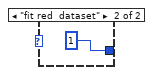
[diagram p14: hidden frame]
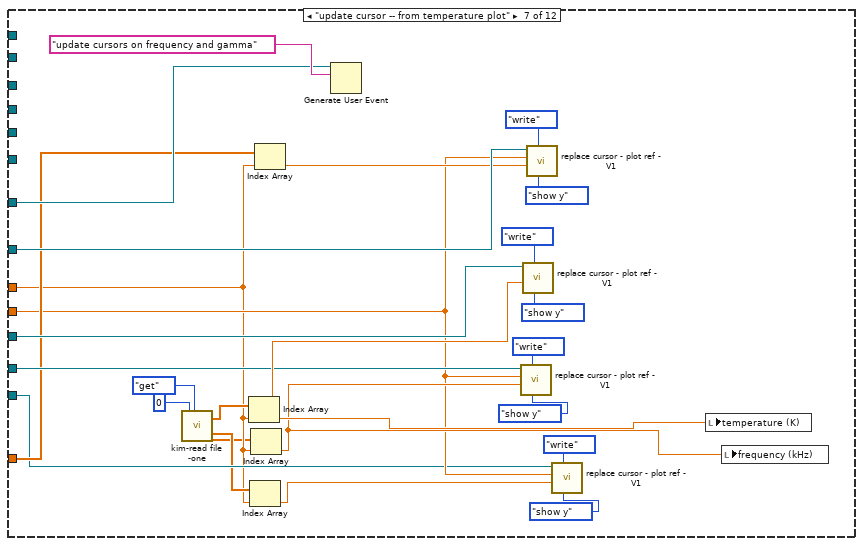
[diagram p15: hidden frame]
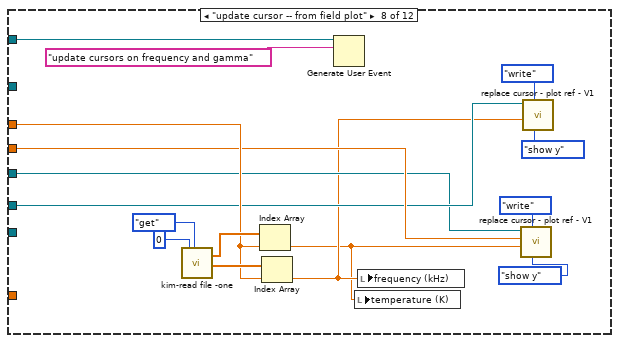
[diagram p16: hidden frame]
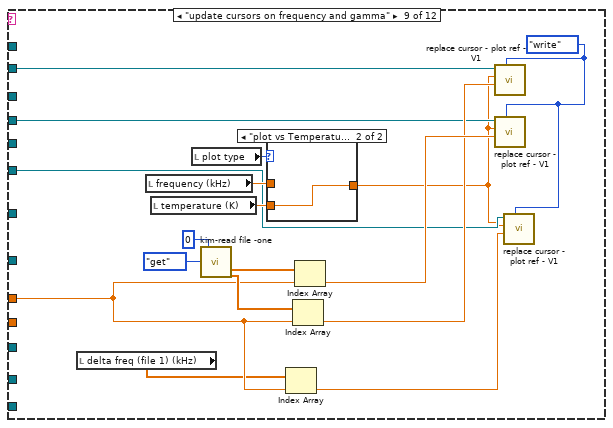
[diagram p17: hidden frame]
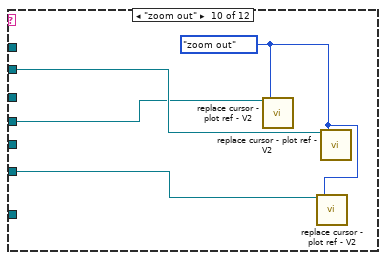
[diagram p19: hidden frame]
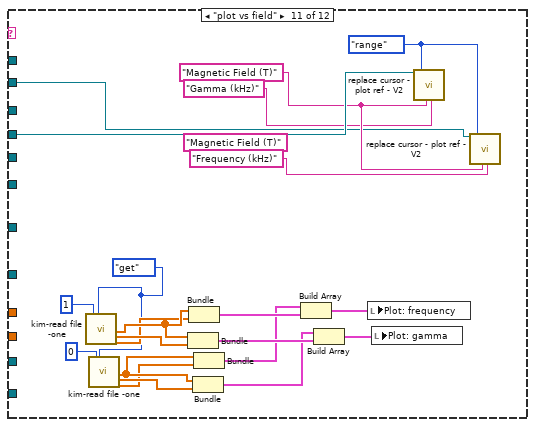
[diagram p20: hidden frame]
diagram:
  w45 = "action"  # user action
  w47 = "action"  # user event
  n1 = control-ref of="Plot: temp vs time"() -> (w19:refnum<vi>)
  n2 = control-ref of="Plot: frequency"() -> (w30:refnum<vi>)
  n3 = control-ref of="Plot: delta freq vs time"() -> (w2:refnum<vi>)
  n4 = Build Array(1, 2, 3) -> (w15:i32[])
  n5 = Build Array(1, 2, 3) -> (w14:i32[])
  n6 = Build Array(1, 2, 3) -> (w4:i32[])
  n7 = Create User Event(user event datatype=w45) -> (user event=w41:refnum<user-event>)  [unwired: 1 in, 1 out]
  n8 = Bundle By Name(cluster=T1 {"left"=0.0, "right "=0.0, "center"=0.0, "window"=0.0, "cursors"=[], "relative"=0, "absolute"=0, "fixed vertical offset"=0.0, "vertical offset"=0.0, "skew"=0.0, "default window frac"=0.0, "kind"=enum."symmetric", "skew.left"=0.0, "skew.right"=0.0, "Plot ref"=refnum, "wing order"=enum."forw"} ("cursor bracket in"), "Plot ref"=w30, "cursors"=w15, "fixed vertical offset"=0.0, "default window frac"=0.3 ("fixed vertical offset"), "kind"=enum16{"symmetric", "skewed", "fancy"}."symmetric") -> (w39:T1)
  n9 = Create User Event(user event datatype=w47) -> (user event=w44:refnum<user-event>)  [unwired: 1 in, 1 out]
  n10 = Bundle By Name(cluster=T1 {"left"=0.0, "right "=0.0, "center"=0.0, "window"=0.0, "cursors"=[], "relative"=0, "absolute"=0, "fixed vertical offset"=0.0, "vertical offset"=0.0, "skew"=0.0, "default window frac"=0.0, "kind"=enum."symmetric", "skew.left"=0.0, "skew.right"=0.0, "Plot ref"=refnum, "wing order"=enum."forw"} ("cursor bracket in"), "Plot ref"=w19, "cursors"=w14, "fixed vertical offset"=0.0, "default window frac"=0.3 ("fixed vertical offset"), "kind"=enum16{"symmetric", "skewed", "fancy"}."skewed") -> (w28:T1)
  n11 = Bundle By Name(cluster=T1 {"left"=0.0, "right "=0.0, "center"=0.0, "window"=0.0, "cursors"=[], "relative"=0, "absolute"=0, "fixed vertical offset"=0.0, "vertical offset"=0.0, "skew"=0.0, "default window frac"=0.0, "kind"=enum."symmetric", "skew.left"=0.0, "skew.right"=0.0, "Plot ref"=refnum, "wing order"=enum."forw"} ("cursor bracket in"), "Plot ref"=w2, "cursors"=w4, "fixed vertical offset"=0.0, "default window frac"=0.3 ("fixed vertical offset"), "kind"=enum16{"symmetric", "skewed", "fancy"}."skewed") -> (w13:T1)
  n12 = register-events(w41) -> (reference out=w46:refnum<event-registration>)  [unwired: 2 in, 1 out]
  n13 = control-ref of="cursor bracket: freq"() -> (w17:refnum<vi>)
  n14 = control-ref of="cursor bracket: delta freq vs time"() -> (w3:refnum<vi>)
  n15 = register-events(w44) -> (reference out=w48:refnum<event-registration>)  [unwired: 2 in, 1 out]
  n16 = control-ref of="cursor bracket: temp vs time"() -> (w16:refnum<vi>)
  n17 = while {
    tunnel: w46 -> [w52]
    tunnel: w41 -> [w49]
    stop <- FALSE stop-if-true
    n18 = event shown="[1] <user action>: User Event" {
      selector: w52 -> [_ _]
      dyn-events: _ -> [_ _]
      timeout: _ -> [_ _]
      tunnel: w49 -> [_ w66]
      event Timeout {
        n19 = event-data() -> ()  [unwired: 1 in, 2 out]
      }
      event User Event {
        n20 = event-data() -> ("user action"=w68:string)  [unwired: 1 in]
        n21 = local read "delta freq (file 1) (kHz)"() -> (w56:dbl[])
        n22 = local read "current index"() -> (w61:dbl)
        n23 = local read "time (min)"() -> (w60:dbl)
        n24 = control-ref of="Plot: frequency"() -> (w64:refnum<vi>)
        n25 = control-ref of="Plot: gamma"() -> (w65:refnum<vi>)
        n26 = control-ref of="Plot: delta frequency"() -> (w59:refnum<vi>)
        n27 = control-ref of="Plot: delta freq vs time"() -> (w57:refnum<vi>)
        n28 = control-ref of="Plot: temp vs time"() -> (w63:refnum<vi>)
        n29 = control-ref of="Plot: freq vs time"() -> (w62:refnum<vi>)
        n30 = control-ref of="Plot: gamma vs time"() -> (w53:refnum<vi>)
        n31 = control-ref of="cursor bracket: delta freq vs time"() -> (w54:refnum<vi>)
        n32 = control-ref of="cursor bracket: temp vs time"() -> (w58:refnum<vi>)
        n33 = control-ref of="cursor bracket: freq"() -> (w55:refnum<vi>)
        n34 = for {
          N: 1 -> [_]
          tunnel: w68 -> [w83]
          tunnel: w66 -> [w82]
          tunnel: w65 -> [w81]
          tunnel: w64 -> [w80]
          tunnel: w63 -> [w79]
          tunnel: w62 -> [w78]
          tunnel: w61 -> [w77]
          tunnel: w60 -> [w76]
          tunnel: w59 -> [w75]
          tunnel: w58 -> [w74]
          tunnel: w57 -> [w73]
          tunnel: w56 -> [w72]
          tunnel: w55 -> [w71]
          tunnel: w54 -> [w70]
          tunnel: w53 -> [w69]
          n35 = case shown="\"plot vs temp\"" w83 {
            tunnel: w82 -> [_ w96 _ _ w213 _ w263 w280 _ _ _ w348]
            tunnel: w81 -> [_ _ w147 _ _ _ _ _ w297 w312 w320 _]
            tunnel: w80 -> [_ _ w144 _ _ _ _ _ w298 w313 w317 _]
            tunnel: w79 -> [_ _ _ _ _ _ w265 w277 _ _ _ w340]
            tunnel: w78 -> [_ _ _ _ _ _ w262 w278 _ _ _ w339]
            tunnel: w77 -> [_ _ _ _ _ _ w251 w282 w293 _ _ _]
            tunnel: w76 -> [_ _ _ _ _ _ w254 w279 _ _ _ _]
            tunnel: w75 -> [_ _ _ _ _ _ _ _ w296 w310 _ _]
            tunnel: w74 -> [_ _ _ _ w212 w243 _ _ _ _ _ _]
            tunnel: w73 -> [_ _ _ _ _ _ w259 _ _ _ _ _]
            tunnel: w72 -> [_ _ _ _ _ _ w258 _ _ _ _ _]
            tunnel: w71 -> [_ _ _ _ _ _ _ _ _ _ _ _]
            tunnel: w70 -> [_ _ _ w179 _ _ _ _ _ _ _ _]
            tunnel: w69 -> [_ _ _ _ _ _ w253 _ _ _ _ _]
            frame "False", Default {
            }
            frame "plot" {
              n36 = call "kim-read file -one.vi"("Numeric Control"=0, "container action"=container_action."get") -> ("Temperature (K) Array"=w91:dbl[], "time (min) array"=w85:dbl[], "Gamma (kHz) Array"=w84:dbl[], "Frequency (kHz) Array"=w88:dbl[])  [unwired: 10 in, 4 out]
              n37 = Bundle("time (min) array"=w85, "Temperature (K) Array"=w91) -> (w93:T12)  [unwired: 1 in]
              n38 = Bundle("time (min) array"=w85, "Frequency (kHz) Array"=w88) -> (w95:T13)  [unwired: 1 in]
              n39 = Bundle("time (min) array"=w85, "Gamma (kHz) Array"=w84) -> (w87:T14)  [unwired: 1 in]
              n40 = case shown="\"plot vs Temperature\"" "plot type" {
                tunnel: w96 -> [w98 w100]
                frame "plot vs Temperature" {
                  n41 = Generate User Event(user event=w98, event data cluster="plot vs temp" ("event data")) -> ()  [unwired: 2 in, 2 out]
                }
                frame "plot vs Magnetic Field" {
                  n42 = Generate User Event(user event=w100, event data cluster="plot vs field" ("event data")) -> ()  [unwired: 2 in, 2 out]
                }
              }
              n43 = Build Array(w93) -> (w92:T15)
              n44 = Build Array(w95) -> (w94:T16)
              n45 = Build Array(w87) -> (w86:T17)
              n46 = local write "Plot: temp vs time"(w92) -> ()
              n47 = local write "Plot: freq vs time"(w94) -> ()
              n48 = local write "Plot: gamma vs time"(w86) -> ()
            }
            frame "plot vs temp" {
              w126 = container_action."get" ("container action")
              w143 = cursor_action."range" ("cursor action")
              w148 = container_action."plot" ("container action")
              n49 = local read "best fit parameters"() -> (w113:dbl[])
              n50 = call "kim-read file -one.vi"("Numeric Control"=1, "container action"=w126) -> ("Temperature (K) Array"=w128:dbl[], "Frequency (kHz) Array"=w129:dbl[])  [unwired: 10 in, 6 out]
              n51 = call "kim-read file -one.vi"("Numeric Control"=0, "container action"=w126) -> ("Temperature (K) Array"=w125:dbl[], "Frequency (kHz) Array"=w123:dbl[])  [unwired: 10 in, 6 out]
              n52 = call "replace cursor - plot ref - V2.vi"("Plot ref in"=w147, "cursor action"=w143, "x-label"="Temperature (K)", "y-label"="Gamma (kHz)") -> ()  [unwired: 13 in, 3 out]
              n53 = call "replace cursor - plot ref - V2.vi"("Plot ref in"=w144, "cursor action"=w143, "x-label"="Temperature (K)", "y-label"="Frequency (kHz)") -> ()  [unwired: 13 in, 3 out]
              n54 = call "fit function selector.vi"("fit using"="fit using", "temperature"=w128, "best fit parameters"=w113) -> ("freq out"=w134:dbl[])  [unwired: 6 in, 2 out]
              n55 = call "fit function selector.vi"("fit using"="fit using", "temperature"=w125, "best fit parameters"=w113) -> ("freq out"=w132:dbl[])  [unwired: 6 in, 2 out]
              n56 = Subtract(x=w123, y=w132) -> (x-y=w131:dbl[])
              n57 = Subtract(x=w129, y=w134) -> (x-y=w133:dbl[])
              n58 = local read "plot type"() -> (w136:T4)
              n59 = local read "fit dataset"() -> (w119:enum16{"fit blue dataset", "fit red  dataset"})
              n60 = Bundle("Temperature (K) Array"=w125, w131) -> (w116:cluster{"Temperature (K) Array":dbl[], dbl[]})  [unwired: 1 in]
              n61 = Bundle("Temperature (K) Array"=w128, w133) -> (w117:cluster{"Temperature (K) Array":dbl[], dbl[]})  [unwired: 1 in]
              n62 = call "kim-read file -one.vi"("Numeric Control"=0) -> ("Temperature (K) Array"=w112:dbl[], "time (min) array"=w110:dbl[], "Frequency (kHz) Array"=w111:dbl[])  [unwired: 11 in, 5 out]
              n63 = case shown="\"fit red  dataset\"" w119 {
                tunnel: [0 ("Numeric Control") 1 ("Numeric Control")] -> w118
                frame "fit blue dataset", Default {
                }
                frame "fit red  dataset" {
                }
              }
              n64 = call "fit function selector.vi"("fit using"="fit using", "temperature"=w112, "best fit parameters"=w113) -> ("freq out"=w114:dbl[])  [unwired: 6 in, 2 out]
              n65 = call "kim-read file -one.vi"("Numeric Control"=1, "plot type"=w136, "container action"=w148) -> ("Plot linew"=w137:T19, "Plot freq"=w138:T20)  [unwired: 9 in, 6 out]
              n66 = call "kim-read file -one.vi"("Numeric Control"=0, "plot type"=w136, "container action"=w148) -> ("Plot linew"=w139:T19, "Plot freq"=w140:T20)  [unwired: 9 in, 6 out]
              n67 = Build Array(w116, w117) -> (→"Plot: delta frequency":cluster{"Temperature (K) Array":dbl[], dbl[]}[])
              n68 = Subtract(x=w111, y=w114) -> (x-y=w109:dbl[])
              "delta freq (file 1) (kHz)" <- w109
              n69 = call "kim-read file -one.vi"("Numeric Control"=w118, "container action"=container_action."get") -> ("Temperature (K) Array"=w121:dbl[])  [unwired: 10 in, 7 out]
              n70 = Bundle("time (min) array"=w110, w109) -> (w108:cluster{"time (min) array":dbl[], dbl[]})  [unwired: 1 in]
              n71 = Build Array(w140, w138) -> (w104:T21)
              n72 = Build Array(w139, w137) -> (w135:T22)
              n73 = call "fit function selector.vi"("fit using"="fit using", "temperature"=w121, "best fit parameters"=w113) -> ("freq out"=w120:dbl[])  [unwired: 6 in, 2 out]
              n74 = Build Array(w108) -> (→"Plot: delta freq vs time":cluster{"time (min) array":dbl[], dbl[]}[])
              n75 = local write "Plot: gamma"(w135) -> ()
              n76 = Bundle("Temperature (K) Array"=w121, "freq out"=w120) -> (w105:T23)  [unwired: 1 in]
              n77 = case shown="False" "plot fit?" {
                tunnel: w105 -> [_ w154]
                tunnel: w104 -> [w151 w153]
                tunnel: [w151 w152] -> w103
                frame False {
                }
                frame True {
                  n78 = Build Array (concatenate)(w153, w154) -> (w152:T7)
                }
              }
              n79 = local write "Plot: frequency"(w103) -> ()
            }
            frame "poor man lockin" {
              w174 = array_transformation_action."nomalize (by abs magn)" ("action")
              w198 = 0.0 ("center x")
              # "temperature"
              # "frequency"
              n80 = call "kim-read file -one.vi"("Numeric Control"=0, "container action"=container_action."get") -> ("Temperature (K) Array"=w184:dbl[], "time (min) array"=w186:dbl[], "Frequency (kHz) Array"=w183:dbl[])  [unwired: 10 in, 5 out]
              n81 = call "cursor window logic V2.vi"("cursor window action"=cursor_window_action."check", "cursor window in"=w179) -> ("cursor window out"=w187:T1)  [unwired: 8 in, 1 out]
              n82 = Unbundle By Name(w187) -> ("window"=w177:dbl)
              "averaging window (min)" <- w177
              n83 = Re/Im To Complex(1:w183, 2:w184) -> (0:w182:cdb[])
              n84 = call "acquire cursor window data.vi"("z in"=w182, "omega in"=w186, "cursor window"=w187) -> ("z out"=w173:cdb[], "omega  out"=w185:dbl[])  [unwired: 4 in, 3 out]
              n85 = call "array transformations V1.vi"("action"=array_transformation_action."remove mean", "array in"=w173) -> ("array out"=w160:cdb[])  [unwired: 9 in]
              n86 = call "Lockin - exponential.vi"("X array (min)"=w185, "Tx (min)"="Lockin wave: Period (min)", "phase"="Lockin wave: Phase", "A"="Lockin wave: Amplitude") -> ("Y array OUT"=w193:cdb[])  [unwired: 7 in]
              n87 = Divide(x=w177, y="Lockin wave: Period (min)") -> (x/y=w176:dbl)
              n88 = call "array transformations V1.vi"("phase"="phase", "action"=array_transformation_action."rotate phase", "array in"=w160) -> ("array out"=w158:cdb[])  [unwired: 8 in]
              n89 = Complex To Re/Im(x + iy=w158) -> (x=w181:dbl[], y=w180:dbl[])
              n90 = Multiply(x=w193, y=w180) -> (x*y=w192:cdb[])
              n91 = Multiply(x=w193, y=w181) -> (x*y=w191:cdb[])
              n92 = call "filter - lockin.vi"("time  in (min)"=w185, "z in"=w191, "time window (min)"=w177) -> ("mean"=w188:cdb)  [unwired: 13 in, 3 out]
              n93 = local write "window/period"(w176) -> ()
              n94 = call "filter - lockin.vi"("time  in (min)"=w185, "z in"=w192, "time window (min)"=w177) -> ("mean"=w189:cdb)  [unwired: 13 in, 3 out]
              n95 = Build Array(w189) -> (w166:cdb[])
              n96 = Build Array(w188) -> (w175:cdb[])
              n97 = Negate(x=w166) -> (-x=w165:cdb[])
              n98 = call "array transformations V1.vi"("action"=w174, "array in"=w175) -> ("array out"=w168:cdb[])  [unwired: 9 in]
              n99 = call "array transformations V1.vi"("action"=w174, "array in"=w165) -> ("array out"=w169:cdb[])  [unwired: 9 in]
              n100 = Index Array(array=w169, index=0) -> (element=w164:cdb)
              n101 = Index Array(array=w168, index=0) -> (element=w167:cdb)
              n102 = Complex To Polar(r * e^(i*theta)=w164) -> (theta=w163:dbl)  [unwired: 1 out]
              "phase of Frequency (rad)" <- w163
              n103 = Complex To Polar(r * e^(i*theta)=w167) -> (theta=w162:dbl)  [unwired: 1 out]
              "phase of Temperature (rad)" <- w162
              n104 = Complex To Re/Im(x + iy=w169) -> (x=w204:dbl[], y=w205:dbl[])
              n105 = Complex To Re/Im(x + iy=w168) -> (x=w202:dbl[], y=w203:dbl[])
              n106 = Subtract(x=w163, y=w162) -> (x-y=→"phase of Frequency vs Temperature phase(rad)":dbl)
              n107 = Bundle(w204, w205) -> (w200:cluster{dbl[], dbl[]})  [unwired: 1 in]
              n108 = Bundle(w202, w203) -> (w190:cluster{dbl[], dbl[]})  [unwired: 1 in]
              n109 = call "draw a circle.vi"("number of points"=10, "center Y"=w198, "center x"=w198, "radius"=1.0) -> ("output cluster"=w201:cluster{dbl[], dbl[]})  [unwired: 7 in]
              n110 = Build Array(w200, w190, w201) -> (→"Plot: lockin":cluster{dbl[], dbl[]}[])
            }
            frame "update fit" {
              (unwired) 1 ("Numeric Control")
              n111 = Generate User Event(user event=w213, event data cluster="plot" ("event data")) -> ()  [unwired: 2 in, 2 out]
              n112 = case shown="\"fit blue dataset\", Default" "fit dataset" {
                tunnel: [0 ("Numeric Control") 1 ("Numeric Control")] -> w221
                frame "fit blue dataset", Default {
                }
                frame "fit red  dataset" {
                }
              }
              n113 = call "cursor window logic V2.vi"("cursor window action"=cursor_window_action."check", "cursor window in"=w212) -> ("cursor window out"=w211:T1)  [unwired: 8 in, 1 out]
              n114 = call "kim-read file -one.vi"("Numeric Control"=w221, "container action"=container_action."get") -> ("Temperature (K) Array"=w217:dbl[], "time (min) array"=w210:dbl[], "Frequency (kHz) Array"=w209:dbl[])  [unwired: 10 in, 5 out]
              n115 = local read "fit using"() -> (w219:T5)
              n116 = call "fit -- freq vs T - V3.vi"("time points"=w210, "fit using"=w219, "temperature points"=w217, "frequency points"=w209, "cursor bracket: freq"=w211) -> ("best fit parameters"=→"best fit parameters":dbl[])  [unwired: 7 in, 3 out]
            }
            frame "update slope" {
              n117 = local read "fit dataset"() -> (w238:enum16{"fit blue dataset", "fit red  dataset"})
              n118 = call "cursor window logic V2.vi"("cursor window action"=cursor_window_action."check", "cursor window in"=w243) -> ("cursor window out"=w242:T1)  [unwired: 8 in, 1 out]
              n119 = case shown="\"fit blue dataset\", Default" w238 {
                tunnel: [0 ("Numeric Control") 1 ("Numeric Control")] -> w246
                frame "fit blue dataset", Default {
                }
                frame "fit red  dataset" {
                }
              }
              n120 = Unbundle By Name(w242) -> ("left"=w232:dbl, "right"=w231:dbl)
              n121 = call "kim-read file -one.vi"("Numeric Control"=w246, "container action"=container_action."get") -> ("Temperature (K) Array"=w234:dbl[], "time (min) array"=w233:dbl[], "Frequency (kHz) Array"=w241:dbl[])  [unwired: 10 in, 5 out]
              n122 = call "get cursor win - ordered - V2.vi"("right"=w231, "left"=w232, "freq"=w241, "time points"=w233) -> ("freq out"=w230:dbl[], "time out"=w225:dbl[])  [unwired: 6 in]
              n123 = call "get cursor win - ordered - V2.vi"("right"=w231, "left"=w232, "freq"=w234, "time points"=w233) -> ("freq out"=w226:dbl[])  [unwired: 6 in, 1 out]
              n124 = call "least square linear interpolation.vi"("X"=w225, "Y"=w226) -> ("slope"=→"slope temp vs time (K/min)":dbl)  [unwired: 8 in, 1 out]
              n125 = call "least square linear interpolation.vi"("X"=w226, "Y"=w230) -> ("slope"=w229:dbl)  [unwired: 8 in, 1 out]
              n126 = call "least square linear interpolation.vi"("X"=w225, "Y"=w230) -> ("slope"=w240:dbl)  [unwired: 8 in, 1 out]
              n127 = Array Size(array=w230) -> (size(s)=w236:i32)
              n128 = Decrement(x=w236) -> (x-1=w235:i32)
              n129 = Index Array(array=w230, index #1=0 ("index"), index #2=w235) -> (element #1=w228:dbl)  [unwired: 1 out]
              n130 = Divide(x=w229, y=w228) -> (x/y=→"slope vs temp (1/K)":dbl)
              n131 = Divide(x=w240, y=w228) -> (x/y=→"slope vs time (1/min)":dbl)
            }
            frame "update cursor -- from temperature plot" {
              n132 = call "kim-read file -one.vi"("Numeric Control"=0, "container action"=container_action."get") -> ("Temperature (K) Array"=w269:dbl[], "Gamma (kHz) Array"=w252:dbl[], "Frequency (kHz) Array"=w249:dbl[])  [unwired: 10 in, 5 out]
              n133 = Index Array(array=w269, index=w251) -> (element=w267:dbl)
              n134 = Index Array(array=w252, index=w251) -> (element=w250:dbl)
              n135 = Index Array(array=w249, index=w251) -> (element=w266:dbl)
              n136 = Index Array(array=w258, index=w251) -> (element=w257:dbl)
              n137 = Generate User Event(user event=w263, event data cluster="update cursors on frequency and gamma" ("event data")) -> ()  [unwired: 2 in, 2 out]
              n138 = call "replace cursor - plot ref - V1.vi"("label"=enum16{"hide", "show x", "show y", "show (x,y)"}."show y", "action"=enum16{"", "read", "write"}."write", "new  Y"=w266, "new X"=w254, "Plot ref in"=w262) -> ()  [unwired: 4 in, 3 out]
              n139 = call "replace cursor - plot ref - V1.vi"("label"=enum16{"hide", "show x", "show y", "show (x,y)"}."show y", "action"=enum16{"", "read", "write"}."write", "new  Y"=w267, "Plot ref in"=w265) -> ()  [unwired: 5 in, 3 out]
              n140 = call "replace cursor - plot ref - V1.vi"("label"=enum16{"hide", "show x", "show y", "show (x,y)"}."show y", "action"=enum16{"", "read", "write"}."write", "new  Y"=w257, "new X"=w254, "Plot ref in"=w259) -> ()  [unwired: 4 in, 3 out]
              n141 = call "replace cursor - plot ref - V1.vi"("label"=enum16{"hide", "show x", "show y", "show (x,y)"}."show y", "action"=enum16{"", "read", "write"}."write", "new  Y"=w250, "new X"=w254, "Plot ref in"=w253) -> ()  [unwired: 4 in, 3 out]
              n142 = local write "temperature (K)"(w267) -> ()
              n143 = local write "frequency (kHz)"(w266) -> ()
            }
            frame "update cursor -- from field plot" {
              n144 = call "kim-read file -one.vi"("Numeric Control"=0, "container action"=container_action."get") -> ("Temperature (K) Array"=w285:dbl[], "Field (T) Array"=w284:dbl[])  [unwired: 10 in, 6 out]
              n145 = Index Array(array=w285, index=w282) -> (element=w275:dbl)
              n146 = Index Array(array=w284, index=w282) -> (element=w276:dbl)
              n147 = Generate User Event(user event=w280, event data cluster="update cursors on frequency and gamma" ("event data")) -> ()  [unwired: 2 in, 2 out]
              n148 = local write "temperature (K)"(w275) -> ()
              n149 = local write "frequency (kHz)"(w276) -> ()
              n150 = call "replace cursor - plot ref - V1.vi"("label"=enum16{"hide", "show x", "show y", "show (x,y)"}."show y", "action"=enum16{"", "read", "write"}."write", "new  Y"=w275, "new X"=w279, "Plot ref in"=w277) -> ()  [unwired: 4 in, 3 out]
              n151 = call "replace cursor - plot ref - V1.vi"("label"=enum16{"hide", "show x", "show y", "show (x,y)"}."show y", "action"=enum16{"", "read", "write"}."write", "new  Y"=w276, "Plot ref in"=w278) -> ()  [unwired: 5 in, 3 out]
            }
            frame "update cursors on frequency and gamma" {
              w295 = enum16{"", "read", "write"}."write" ("action")
              n152 = local read "delta freq (file 1) (kHz)"() -> (w292:dbl[])
              n153 = local read "frequency (kHz)"() -> (w301:dbl)
              n154 = local read "temperature (K)"() -> (w300:dbl)
              n155 = local read "plot type"() -> (w299:T4)
              n156 = call "kim-read file -one.vi"("Numeric Control"=0, "container action"=container_action."get") -> ("Gamma (kHz) Array"=w307:dbl[], "Frequency (kHz) Array"=w304:dbl[])  [unwired: 10 in, 6 out]
              n157 = case shown="\"plot vs Temperature\"" w299 {
                tunnel: [w308 w309] -> w294
                tunnel: w300 -> [_ w309]
                tunnel: w301 -> [w308 _]
                frame "plot vs Magnetic Field", Default {
                }
                frame "plot vs Temperature" {
                }
              }
              n158 = Index Array(array=w292, index=w293) -> (element=w291:dbl)
              n159 = Index Array(array=w304, index=w293) -> (element=w305:dbl)
              n160 = Index Array(array=w307, index=w293) -> (element=w306:dbl)
              n161 = call "replace cursor - plot ref - V1.vi"("action"=w295, "new  Y"=w305, "new X"=w294, "Plot ref in"=w298) -> ()  [unwired: 5 in, 3 out]
              n162 = call "replace cursor - plot ref - V1.vi"("action"=w295, "new  Y"=w306, "new X"=w294, "Plot ref in"=w297) -> ()  [unwired: 5 in, 3 out]
              n163 = call "replace cursor - plot ref - V1.vi"("action"=w295, "new  Y"=w291, "new X"=w294, "Plot ref in"=w296) -> ()  [unwired: 5 in, 3 out]
            }
            frame "zoom out" {
              w311 = cursor_action."zoom out" ("cursor action")
              n164 = call "replace cursor - plot ref - V2.vi"("Plot ref in"=w312, "cursor action"=w311) -> ()  [unwired: 15 in, 3 out]
              n165 = call "replace cursor - plot ref - V2.vi"("Plot ref in"=w310, "cursor action"=w311) -> ()  [unwired: 15 in, 3 out]
              n166 = call "replace cursor - plot ref - V2.vi"("Plot ref in"=w313, "cursor action"=w311) -> ()  [unwired: 15 in, 3 out]
            }
            frame "plot vs field" {
              w321 = cursor_action."range" ("cursor action")
              w322 = container_action."get" ("container action")
              (unwired) "Magnetic Field (T)"
              w319 = "Magnetic Field (T)"
              n167 = call "kim-read file -one.vi"("Numeric Control"=1, "container action"=w322) -> ("Field (T) Array"=w328:dbl[], "Gamma (kHz) Array"=w327:dbl[], "Frequency (kHz) Array"=w326:dbl[])  [unwired: 10 in, 5 out]
              n168 = call "kim-read file -one.vi"("Numeric Control"=0, "container action"=w322) -> ("Field (T) Array"=w325:dbl[], "Gamma (kHz) Array"=w324:dbl[], "Frequency (kHz) Array"=w323:dbl[])  [unwired: 10 in, 5 out]
              n169 = Bundle("Field (T) Array"=w328, "Gamma (kHz) Array"=w327) -> (w333:T24)  [unwired: 1 in]
              n170 = Bundle("Field (T) Array"=w328, "Frequency (kHz) Array"=w326) -> (w334:T25)  [unwired: 1 in]
              n171 = Bundle("Field (T) Array"=w325, "Gamma (kHz) Array"=w324) -> (w314:T24)  [unwired: 1 in]
              n172 = Bundle("Field (T) Array"=w325, "Frequency (kHz) Array"=w323) -> (w315:T25)  [unwired: 1 in]
              n173 = Build Array(w315, w334) -> (w331:T26)
              n174 = Build Array(w314, w333) -> (w332:T27)
              n175 = local write "Plot: frequency"(w331) -> ()
              n176 = local write "Plot: gamma"(w332) -> ()
              n177 = call "replace cursor - plot ref - V2.vi"("Plot ref in"=w320, "cursor action"=w321, "x-label"=w319, "y-label"="Gamma (kHz)") -> ()  [unwired: 13 in, 3 out]
              n178 = call "replace cursor - plot ref - V2.vi"("Plot ref in"=w317, "cursor action"=w321, "x-label"=w319, "y-label"="Frequency (kHz)") -> ()  [unwired: 13 in, 3 out]
            }
            frame "read file" {
              w343 = container_action."read file" ("container action")
              w338 = cursor_action."range" ("cursor action")
              n179 = local read "file 1 path"() -> (w341:path)
              n180 = local read "file 2 path"() -> (w342:path)
              n181 = call "kim-read file -one.vi"("File Path Control"=w342, "Numeric Control"=1, "container action"=w343) -> ("OK?"=→"file 2 -- OK":bool)  [unwired: 9 in, 7 out]
              n182 = call "kim-read file -one.vi"("File Path Control"=w341, "Numeric Control"=0, "container action"=w343) -> ("OK?"=w346:bool)  [unwired: 9 in, 7 out]
              "file 1 -- OK" <- w346
              n183 = call "replace cursor - plot ref - V2.vi"("Plot ref in"=w340, "cursor action"=w338, "y-label"="Temperature (K)" ("x-label")) -> ()  [unwired: 14 in, 3 out]
              n184 = case shown="True" w346 {
                tunnel: w348 -> [_ w349]
                frame False {
                }
                frame True {
                  n185 = Generate User Event(user event=w349, event data cluster="plot" ("event data")) -> ()  [unwired: 2 in, 2 out]
                }
              }
              n186 = call "replace cursor - plot ref - V2.vi"("Plot ref in"=w339, "cursor action"=w338, "x-label"="Time (min)", "y-label"="Frequency (kHz)" ("x-label")) -> ()  [unwired: 13 in, 3 out]
            }
          }
        }
      }
    }
    n187 = Wait (ms)(milliseconds to wait=u32 1) -> ()  [unwired: 1 out]
  }
  n188 = call "cursor window logic V2.vi"("cursor window action"=cursor_window_action."init", "cursor window in"=w17, "cursor window init"=w39) -> ("cursor window out"=w29:refnum<vi>)  [unwired: 7 in, 1 out]
  n189 = call "cursor window logic V2.vi"("cursor window action"=cursor_window_action."init", "cursor window in"=w16, "cursor window init"=w28) -> ("cursor window out"=w18:refnum<vi>)  [unwired: 7 in, 1 out]
  n190 = call "cursor window logic V2.vi"("cursor window action"=cursor_window_action."init", "cursor window in"=w3, "cursor window init"=w13) -> ("cursor window out"=w1:refnum<vi>)  [unwired: 7 in, 1 out]
  n191 = while {
    tunnel: w48 -> [w374]
    tunnel: w41 -> [w371]
    tunnel: w44 -> [w367]
    tunnel: w29 -> [_]
    tunnel: w18 -> [_]
    tunnel: w1 -> [_]
    stop <- FALSE stop-if-true
    n192 = control-ref of="Plot: lockin"() -> (w351:refnum<vi>)
    n193 = local read "current index"() -> (w365:dbl)
    n194 = control-ref of="Plot: lockin"() -> (w353:refnum<vi>)
    n195 = control-ref of="Plot: frequency"() -> (w369:refnum<vi>)
    n196 = control-ref of="Plot: temp vs time"() -> (w366:refnum<vi>)
    n197 = control-ref of="Plot: freq vs time"() -> (w370:refnum<vi>)
    n198 = control-ref of="Plot: gamma"() -> (w368:refnum<vi>)
    n199 = control-ref of="Plot: delta frequency"() -> (w356:refnum<vi>)
    n200 = control-ref of="Plot: delta freq vs time"() -> (w354:refnum<vi>)
    n201 = control-ref of="cursor bracket: delta freq vs time"() -> (w352:refnum<vi>)
    n202 = control-ref of="file 1"() -> (w362:refnum<vi>)
    n203 = control-ref of="file 2"() -> (w361:refnum<vi>)
    n204 = control-ref of="cursor bracket: temp vs time"() -> (w357:refnum<vi>)
    n205 = control-ref of="cursor bracket: freq"() -> (w355:refnum<vi>)
    n206 = control-ref of="sweep folder 1"() -> (w358:refnum<vi>)
    n207 = control-ref of="sweep folder 2"() -> (w359:refnum<vi>)
    n208 = event shown="[1] Key Down" {
      selector: w374 -> [_ _ _ _ _ _ _ _ _ _ _ _ _ _ _ _ _ _ _ _ _ _ _ _ _ _]
      dyn-events: _ -> [_ _ _ _ _ _ _ _ _ _ _ _ _ _ _ _ _ _ _ _ _ _ _ _ _ _]
      timeout: _ -> [_ _ _ _ _ _ _ _ _ _ _ _ _ _ _ _ _ _ _ _ _ _ _ _ _ _]
      tunnel: [_ _ _ _ _ "plot (p)" _ _ _ _ _ _ _ _ _ _ _ "open (o)" _ _ _ "lockin (l)" _ _ _ _] -> _
      tunnel: w371 -> [_ w392 w493 _ w506 w510 w511 w516 _ w669 w678 _ w715 _ _ _ w731 w736 _ _ _ w882 w886 w888 _ w901]
      tunnel: w370 -> [_ w388 _ _ _ _ _ _ w662 _ _ _ _ _ _ _ _ _ _ _ _ _ _ _ _ _]
      tunnel: w369 -> [_ w387 _ _ _ _ _ w521 _ _ _ _ _ _ _ _ _ _ _ _ _ _ _ _ _ _]
      tunnel: w368 -> [_ w386 _ _ _ _ _ w520 _ _ _ _ _ _ _ _ _ _ _ _ _ _ _ _ _ _]
      tunnel: w367 -> [_ w379 _ _ _ _ _ _ w668 _ _ _ _ w719 w723 _ _ _ _ w749 _ _ _ _ _ _]
      tunnel: w366 -> [_ w389 _ _ _ _ _ _ _ _ w680 _ _ _ _ _ _ _ _ _ _ _ _ _ _ _]
      tunnel: w365 -> [_ _ _ _ _ _ _ w518 _ _ _ _ _ _ _ _ _ _ _ _ _ _ _ _ _ _]
      tunnel: w362 -> [_ w381 _ _ _ _ _ w517 _ _ _ w713 w718 _ _ _ _ _ _ _ _ _ _ _ _ _]
      tunnel: w361 -> [_ w380 _ _ _ _ _ w513 _ _ _ _ _ _ _ w726 w730 _ _ _ _ _ _ _ _ _]
      tunnel: "folder 1" -> [_ _ _ _ _ _ _ w515 _ _ _ w710 _ _ _ _ _ _ _ _ _ _ _ _ _ _]
      tunnel: "folder 2" -> [_ _ _ _ _ _ _ w514 _ _ _ _ _ _ _ w725 _ _ _ _ _ _ _ _ _ _]
      tunnel: "main folder" -> [_ _ _ _ _ _ _ _ _ _ _ _ _ _ _ _ _ _ w740 w752 _ _ _ _ _ _]
      tunnel: w359 -> [_ _ _ _ _ _ _ _ _ _ _ _ _ _ _ _ _ _ _ _ _ _ _ _ _ _]
      tunnel: w358 -> [_ _ _ _ _ _ _ _ _ _ _ _ _ _ _ _ _ _ _ _ _ _ _ _ _ _]
      tunnel: w355 -> [_ w391 _ _ _ _ _ _ _ _ w676 _ _ _ _ _ _ _ _ _ w876 _ _ _ _ _]
      tunnel: w357 -> [_ w390 _ _ _ _ _ _ _ _ w677 _ _ _ _ _ _ _ _ _ _ _ _ w890 _ _]
      tunnel: w356 -> [_ w385 _ _ _ _ _ _ _ _ _ _ _ _ _ _ _ _ _ _ _ _ _ _ _ _]
      tunnel: w354 -> [_ w378 _ _ _ _ _ _ _ _ _ _ _ _ _ _ _ _ _ _ _ _ _ _ _ _]
      tunnel: w353 -> [_ w377 _ _ _ _ _ _ _ w675 _ _ _ _ _ _ _ _ _ _ _ _ _ _ _ _]
      tunnel: w352 -> [_ w376 w495 w505 _ _ _ _ _ _ _ _ _ _ _ _ _ _ _ _ _ _ _ _ _ _]
      tunnel: w351 -> [_ w375 _ _ _ _ _ _ _ _ _ _ _ _ _ _ _ _ _ _ _ _ _ _ _ _]
      event Timeout {
        n209 = event-data() -> ()  [unwired: 1 in, 2 out]
      }
      event Key Down {
        n210 = event-data() -> ("Char"=w384:i16, "VKey"=w393:T6)  [unwired: 1 in]
        "Char" <- w384
        "VKey" <- w393
        n211 = Build Array(w384) -> (w383:i16[])
        n212 = Byte Array To String(unsigned byte array=w383) -> (string=w382:string)
        n213 = case shown="\"ASCII\", Default" w393 {
          selector: w393 -> [_ w437 _ _ w480]
          tunnel: w384 -> [_ _ _ _ _]
          tunnel: w392 -> [w402 w445 _ _ w477]
          tunnel: w391 -> [w401 w444 _ _ _]
          tunnel: w390 -> [w400 w443 _ _ w476]
          tunnel: w387 -> [_ _ w470 _ _]
          tunnel: w389 -> [_ _ w469 _ _]
          tunnel: w388 -> [_ _ w468 _ _]
          tunnel: w386 -> [_ _ w467 _ _]
          tunnel: w385 -> [_ _ w462 _ _]
          tunnel: w382 -> [w399 _ _ _ _]
          tunnel: w381 -> [w398 w442 _ _ _]
          tunnel: w380 -> [w397 w441 _ _ _]
          tunnel: w379 -> [w396 w440 _ _ _]
          tunnel: w378 -> [_ _ w461 _ _]
          tunnel: w377 -> [_ _ w460 _ _]
          tunnel: w376 -> [w395 w439 _ _ _]
          tunnel: w375 -> [w394 w438 _ _ _]
          frame "ASCII", Default {
            n214 = case shown="\" \"" w399 {
              tunnel: w402 -> [_ w403 w405 w408 w409 w411 w413 _ _ w435]
              tunnel: w401 -> [_ _ _ _ _ _ _ _ w432 _]
              tunnel: w400 -> [_ _ _ _ _ _ _ _ w431 _]
              tunnel: w398 -> [_ _ _ _ _ _ _ w417 _ _]
              tunnel: w397 -> [_ _ _ _ _ _ _ w416 _ _]
              tunnel: w396 -> [_ _ _ _ _ _ _ w415 _ _]
              tunnel: w395 -> [_ _ _ _ _ _ _ _ w429 _]
              tunnel: w394 -> [_ _ _ _ _ _ _ _ w428 _]
              frame "0", Default {
              }
              frame "p" {
                # "p"
                n215 = Generate User Event(user event=w403, event data cluster="plot" ("event data")) -> ()  [unwired: 2 in, 2 out]
              }
              frame "o" {
                # "<space>"
                # "o"
                n216 = Generate User Event(user event=w405, event data cluster="read file" ("event data")) -> ()  [unwired: 2 in, 2 out]
              }
              frame " " {
                (unwired) "read file" ("event data")
                # "<space>"
                n217 = Generate User Event(user event=w408, event data cluster="zoom out" ("event data")) -> ()  [unwired: 2 in, 2 out]
              }
              frame "s" {
                n218 = Generate User Event(user event=w409, event data cluster="update slope" ("event data")) -> ()  [unwired: 2 in, 2 out]
              }
              frame "t" {
                n219 = Generate User Event(user event=w411, event data cluster="update fit" ("event data")) -> ()  [unwired: 2 in, 2 out]
              }
              frame "z" {
                # "z"
                n220 = Generate User Event(user event=w413, event data cluster="zoom out" ("event data")) -> ()  [unwired: 2 in, 2 out]
              }
              frame "a" {
                n221 = disable-structure shown="Disabled" {
                  disable-tunnel: w417 -> [w424 _]
                  disable-tunnel: w416 -> [w423 _]
                  disable-tunnel: w415 -> [w418 _]
                  frame Disabled {
                    w422 = save-read_action."increment read from" ("action")
                    (unwired) "read file" ("event data")
                    n222 = call "freq file -- file select controller.vi"("action"=w422, "file select ref"=w423) -> ()  [unwired: 7 in, 3 out]
                    n223 = call "freq file -- file select controller.vi"("action"=w422, "file select ref"=w424) -> ()  [unwired: 7 in, 3 out]
                    n224 = Generate User Event(user event=w418, event data cluster="update file path 1" ("event data")) -> (user event out=w420:refnum<user-event>)  [unwired: 2 in, 1 out]
                    n225 = Generate User Event(user event=w420, event data cluster="update file path 2" ("event data")) -> ()  [unwired: 2 in, 2 out]
                  }
                  frame Enabled {
                  }
                }
              }
              frame "c" {
                # "c"
                n226 = call "replace cursor - plot ref - V2.vi"("Plot ref in"=w428, "new X"=0.0, "new  Y"=0.0, "cursor action"=cursor_action."write") -> ()  [unwired: 13 in, 3 out]
                n227 = call "cursor window logic V2.vi"("cursor window action"=cursor_window_action."check", "cursor window in"=w429) -> ()  [unwired: 8 in, 2 out]
                n228 = call "cursor window logic V2.vi"("cursor window action"=cursor_window_action."check", "cursor window in"=w431) -> ()  [unwired: 8 in, 2 out]
                n229 = call "cursor window logic V2.vi"("cursor window action"=cursor_window_action."check", "cursor window in"=w432) -> ()  [unwired: 8 in, 2 out]
              }
              frame "l" {
                n230 = Generate User Event(user event=w435, event data cluster="poor man lockin" ("event data")) -> ()  [unwired: 2 in, 2 out]
              }
            }
          }
          frame "PageUp", "PageDown" {
            n231 = case shown="\"PageDown\"" w437 {
              tunnel: w445 -> [_ _]
              tunnel: w444 -> [_ _]
              tunnel: w443 -> [_ _]
              tunnel: w442 -> [w452 w459]
              tunnel: w441 -> [w451 w458]
              tunnel: w440 -> [w446 w453]
              tunnel: w439 -> [_ _]
              tunnel: w438 -> [_ _]
              frame "PageUp", Default {
                w450 = save-read_action."increment read from" ("action")
                (unwired) "read file" ("event data")
                n232 = call "freq file -- file select controller.vi"("action"=w450, "file select ref"=w451) -> ()  [unwired: 7 in, 3 out]
                n233 = call "freq file -- file select controller.vi"("action"=w450, "file select ref"=w452) -> ()  [unwired: 7 in, 3 out]
                n234 = Generate User Event(user event=w446, event data cluster="update file path 1" ("event data")) -> (user event out=w448:refnum<user-event>)  [unwired: 2 in, 1 out]
                n235 = Generate User Event(user event=w448, event data cluster="update file path 2" ("event data")) -> ()  [unwired: 2 in, 2 out]
              }
              frame "PageDown" {
                w457 = save-read_action."decrement read from" ("action")
                (unwired) "read file" ("event data")
                n236 = call "freq file -- file select controller.vi"("action"=w457, "file select ref"=w458) -> ()  [unwired: 7 in, 3 out]
                n237 = call "freq file -- file select controller.vi"("action"=w457, "file select ref"=w459) -> ()  [unwired: 7 in, 3 out]
                n238 = Generate User Event(user event=w453, event data cluster="update file path 1" ("event data")) -> (user event out=w455:refnum<user-event>)  [unwired: 2 in, 1 out]
                n239 = Generate User Event(user event=w455, event data cluster="update file path 2" ("event data")) -> ()  [unwired: 2 in, 2 out]
              }
            }
          }
          frame "Escape" {
            n240 = Build Array(w470, w469, w468, w467, w462, w461, w460) -> (w466:refnum<vi>[])
            n241 = for {
              tunnel: w466 -> [w475] mode=indexing
              tunnel: [w474] -> w465
              tunnel: [w473] -> w463 mode=indexing
              n242 = property class="XYGraph (strict)"(reference=w475) -> (reference out=w473:refnum<vi>, "Palette Visible"=w474:bool)  [unwired: 1 in, 1 out]
            }
            n243 = Not(x=w465) -> (.not. x?=w464:bool)
            n244 = for {
              tunnel: w464 -> [w472]
              tunnel: w463 -> [w471] mode=indexing
              n245 = property class="XYGraph (strict)"(reference=w471, "Palette Visible"=w472) -> ()  [unwired: 1 in, 2 out]
            }
          }
          frame "Enter" {
          }
          frame "Up".."Right" {
            n246 = case shown="\"Down\"" w480 {
              tunnel: w476 -> [w482 w485 w488 w491]
              tunnel: [w481 w484 w487 w490] -> w478
              tunnel: w477 -> [w481 w484 w487 w490]
              frame "Up", Default {
                n247 = call "cursor window logic V2.vi"("cursor window action"=cursor_window_action."broaden", "cursor window in"=w482) -> ()  [unwired: 8 in, 2 out]
              }
              frame "Down" {
                n248 = call "cursor window logic V2.vi"("cursor window action"=cursor_window_action."shrink", "cursor window in"=w485) -> ()  [unwired: 8 in, 2 out]
              }
              frame "Left" {
                n249 = call "cursor window logic V2.vi"("cursor window action"=cursor_window_action."move left", "cursor window in"=w488) -> ()  [unwired: 8 in, 2 out]
              }
              frame "Right" {
                n250 = call "cursor window logic V2.vi"("cursor window action"=cursor_window_action."move right", "cursor window in"=w491) -> ()  [unwired: 8 in, 2 out]
              }
            }
            n251 = Generate User Event(user event=w478, event data cluster="update slope" ("event data")) -> ()  [unwired: 2 in, 2 out]
          }
        }
      }
      event "Plot: delta freq vs time": Cursor Move {
        n252 = event-data() -> ("CursIdx"=w494:i32)  [unwired: 1 in]
        n253 = case shown="1..3" w494 {
          selector: w494 -> [_ w498]
          tunnel: w495 -> [_ w500]
          tunnel: w493 -> [_ w496]
          frame 0, Default {
          }
          frame 1..3 {
            n254 = call "cursor window logic V2.vi"("CursIdx"=w498, "cursor window action"=cursor_window_action."cursor moves", "cursor window in"=w500) -> ()  [unwired: 7 in, 2 out]
            n255 = Generate User Event(user event=w496, event data cluster="poor man lockin" ("event data")) -> ()  [unwired: 2 in, 2 out]
          }
        }
      }
      event "window/period": Value Change {
        n256 = event-data() -> ("NewVal"=w502:dbl)  [unwired: 1 in]
        n257 = local read "Lockin wave: Period (min)"() -> (w503:dbl)
        n258 = Multiply(x=w502, y=w503) -> (x*y=w501:dbl)
        n259 = call "cursor window logic V2.vi"("cursor window action"=cursor_window_action."change window", "window"=w501, "cursor window in"=w505) -> ()  [unwired: 7 in, 2 out]
      }
      event "file 1 path", "file 2 path": Value Change {
        n260 = event-data() -> ()  [unwired: 1 in, 1 out]
        n261 = Generate User Event(user event=w506, event data cluster="read file" ("event data")) -> ()  [unwired: 2 in, 2 out]
      }
      event "plot (p)": Value Change {
        n262 = event-data() -> ()  [unwired: 1 in, 2 out]
        n263 = Generate User Event(user event=w510, event data cluster="plot" ("event data")) -> ()  [unwired: 2 in, 2 out]
      }
      event "plot type": Value Change {
        n264 = event-data() -> ()  [unwired: 1 in, 1 out]
        n265 = Generate User Event(user event=w511, event data cluster="plot" ("event data")) -> ()  [unwired: 2 in, 2 out]
      }
      event User Event {
        n266 = event-data() -> ("user event"=w519:string)  [unwired: 1 in]
        n267 = case shown="\"update file path 1\", \"update file path 2\"" w519 {
          selector: w519 -> [_ w525]
          tunnel: w521 -> [_ _]
          tunnel: w520 -> [_ _]
          tunnel: w518 -> [_ _]
          tunnel: w517 -> [_ w531]
          tunnel: w516 -> [_ w530]
          tunnel: w515 -> [_ w529]
          tunnel: w514 -> [_ _]
          tunnel: w513 -> [_ _]
          frame "False", Default {
          }
          frame "update file path 1", "update file path 2" {
            n268 = call "freq file -- file select controller.vi"("action"=save-read_action."copy read from read ring", "file select ref"=w531) -> ("file select OUT"=w539:T2)  [unwired: 7 in, 2 out]
            n269 = Unbundle By Name(w539) -> ("from file"=w535:string, "folder kind"=w534:T3)
            n270 = xnode "Match Regular Expression"("input string"=w525, "regular expression"=".*?(\\d+)") -> ("submatch 1"=w523:string)  [unwired: 4 in, 5 out]
            n271 = call "freq file -- file type selector.vi"("folder kind"=w534, "Sweep folder path"=w529) -> ("folder path"=w533:path, "OK"=w527:bool)  [unwired: 7 in, 1 out]
            n272 = Decimal String To Number(string=w523) -> (number=w522:i32)  [unwired: 2 in, 1 out]
            n273 = Concatenate Strings(w535, ".dat" ("name or relative path")) -> (w538:string)
            n274 = Build Path(base path=w533, name or relative path=w538) -> (appended path=w536:path)
            n275 = call <vilib>:"Check if File or Folder Exists.vi"("path"=w536) -> ("file or folder exists?"=w528:bool, "dup path"=w532:path)  [unwired: 8 in, 1 out]
            n276 = And(x=w527, y=w528) -> (x .and. y?=w526:bool)
            n277 = case shown="True" w526 {
              tunnel: w532 -> [_ w655]
              tunnel: w530 -> [_ w656]
              tunnel: w522 -> [_ w654]
              frame False {
              }
              frame True {
                n278 = case shown="1, Default" w654 {
                  tunnel: w655 -> [w658 w659]
                  frame 1, Default {
                    n279 = local write "file 1 path"(w658) -> ()
                  }
                  frame 2 {
                    n280 = local write "file 2 path"(w659) -> ()
                  }
                }
                n281 = Generate User Event(user event=w656, event data cluster="read file" ("event data")) -> ()  [unwired: 2 in, 2 out]
              }
            }
          }
        }
      }
      event "Plot: freq vs time": Cursor Move {
        n282 = event-data() -> ()  [unwired: 1 in, 5 out]
        n283 = call "replace cursor - plot ref - V2.vi"("Plot ref in"=w662, "cursor action"=cursor_action."read") -> ("read X"=w660:dbl)  [unwired: 15 in, 2 out]
        n284 = call "kim-read file -one.vi"("Numeric Control"=0, "container action"=container_action."get") -> ("time (min) array"=w665:dbl[])  [unwired: 10 in, 7 out]
        n285 = Threshold 1D Array(2:w660, 3:w665) -> (0:w667:dbl)  [unwired: 1 in]
        n286 = local write "current index"(w667) -> ()
        n287 = local write "time (min)"(w660) -> ()
        n288 = Generate User Event(user event=w668, event data cluster="update cursor -- from field plot " ("event data")) -> ()  [unwired: 2 in, 2 out]
      }
      event "Plot: lockin": Cursor Move {
        n289 = event-data() -> ()  [unwired: 1 in, 4 out]
        n290 = call "replace cursor - plot ref - V2.vi"("Plot ref in"=w675, "cursor action"=cursor_action."read") -> ("read X"=w673:dbl, "read Y"=w672:dbl)  [unwired: 15 in, 1 out]
        n291 = Re/Im To Polar(2:w672, 3:w673) -> (0:w671:dbl)  [unwired: 1 out]
        n292 = Generate User Event(user event=w669, event data cluster="poor man lockin" ("event data")) -> ()  [unwired: 2 in, 2 out]
        n293 = local write "phase"(w671) -> ()
      }
      event "Plot: temp vs time": Cursor Move {
        n294 = event-data() -> ("CursIdx"=w679:i32)  [unwired: 1 in]
        n295 = case shown="0" w679 {
          selector: w679 -> [w683 _]
          tunnel: w680 -> [_ w706]
          tunnel: w678 -> [_ w701]
          tunnel: w677 -> [w681 _]
          tunnel: w676 -> [w682 _]
          frame 1..3, Default {
            n296 = call "cursor window logic V2.vi"("CursIdx"=w683, "cursor window action"=cursor_window_action."cursor moves", "cursor window in"=w681) -> ("cursor window out"=w698:T1)  [unwired: 7 in, 1 out]
            n297 = Unbundle By Name(w698) -> ("left"=w695:dbl, "right"=w693:dbl)
            n298 = call "kim-read file -one.vi"("Numeric Control"=0, "container action"=container_action."get") -> ("Temperature (K) Array"=w690:dbl[], "time (min) array"=w694:dbl[])  [unwired: 10 in, 6 out]
            n299 = Threshold 1D Array(2:w693, 3:w694) -> (0:w691:dbl)  [unwired: 1 in]
            n300 = Threshold 1D Array(2:w695, 3:w694) -> (0:w692:dbl)  [unwired: 1 in]
            n301 = Index Array(array=w690, index #1=w692, index #2=w691) -> (element #1=w689:dbl, element #2=w688:dbl)
            n302 = call "Q -- range multiplier -- real.vi"("factor"=1.0, "lower"=w689, "upper"=w688) -> ("center"=w684:dbl, "window"=w686:dbl)  [unwired: 5 in, 2 out]
            n303 = Absolute Value(x=w686) -> (abs(x)=w685:dbl)
            n304 = call "cursor window logic V2.vi"("cursor window action"=cursor_window_action."change cen&win", "window"=w685, "center"=w684, "cursor window in"=w682) -> ()  [unwired: 6 in, 2 out]
          }
          frame 0 {
            n305 = call "replace cursor - plot ref - V1.vi"("action"=enum16{"", "read", "write"}."read", "Plot ref in"=w706) -> ("read X"=w708:dbl)  [unwired: 7 in, 2 out]
            n306 = call "kim-read file -one.vi"("Numeric Control"=0, "container action"=container_action."get") -> ("time (min) array"=w704:dbl[])  [unwired: 10 in, 7 out]
            n307 = Threshold 1D Array(2:w708, 3:w704) -> (0:w707:dbl)  [unwired: 1 in]
            n308 = local write "current index"(w707) -> ()
            n309 = local write "time (min)"(w708) -> ()
            n310 = Generate User Event(user event=w701, event data cluster="update cursor -- from temperature plot" ("event data")) -> ()  [unwired: 2 in, 2 out]
          }
        }
      }
      event Mouse Enter {
        n311 = event-data() -> ()  [unwired: 1 in, 1 out]
        n312 = call "freq file -- file select controller.vi"("Sweep folder path"=w710, "action"=save-read_action."update read list", "file select ref"=w713) -> ("file select ref out"=w711:refnum<vi>)  [unwired: 6 in, 2 out]
        n313 = call "freq file -- file select controller.vi"("action"=save-read_action."copy read from read ring", "file select ref"=w711) -> ()  [unwired: 7 in, 3 out]
      }
      event Value Change {
        n314 = event-data() -> ()  [unwired: 1 in, 1 out]
        n315 = call "freq file -- file select controller.vi"("action"=save-read_action."read event", "file select ref"=w718) -> ()  [unwired: 7 in, 3 out]
        n316 = Generate User Event(user event=w715, event data cluster="read file" ("event data")) -> ()  [unwired: 2 in, 2 out]
      }
      event Value Change; Mouse Down {
        n317 = event-data() -> ()  [unwired: 1 in, 1 out]
        n318 = Generate User Event(user event=w719, event data cluster="update file path 1" ("event data")) -> ()  [unwired: 2 in, 2 out]
      }
      event Value Change; Mouse Down {
        n319 = event-data() -> ()  [unwired: 1 in, 2 out]
        n320 = Generate User Event(user event=w723, event data cluster="update file path 2" ("event data")) -> (user event out=w721:refnum<user-event>)  [unwired: 2 in, 1 out]
        n321 = Generate User Event(user event=w721, event data cluster="update file path 1" ("event data")) -> ()  [unwired: 2 in, 2 out]
      }
      event Mouse Enter {
        n322 = event-data() -> ()  [unwired: 1 in, 4 out]
        n323 = call "freq file -- file select controller.vi"("Sweep folder path"=w725, "action"=save-read_action."update read list", "file select ref"=w726) -> ("file select ref out"=w727:refnum<vi>)  [unwired: 6 in, 2 out]
        n324 = call "freq file -- file select controller.vi"("action"=save-read_action."copy read from read ring", "file select ref"=w727) -> ()  [unwired: 7 in, 3 out]
      }
      event Value Change {
        n325 = event-data() -> ()  [unwired: 1 in, 1 out]
        n326 = call "freq file -- file select controller.vi"("action"=save-read_action."read event", "file select ref"=w730) -> ()  [unwired: 7 in, 3 out]
        n327 = Generate User Event(user event=w731, event data cluster="read file" ("event data")) -> ()  [unwired: 2 in, 2 out]
      }
      event "open (o)": Value Change {
        n328 = event-data() -> ()  [unwired: 1 in, 2 out]
        n329 = Generate User Event(user event=w736, event data cluster="read file" ("event data")) -> ()  [unwired: 2 in, 2 out]
      }
      event "sweep folder 2", "sweep folder 1": Mouse Enter {
        (unwired) TRUE ("Numeric sort?")
        n330 = event-data() -> ("CtlRef"=w737:refnum<vi>)  [unwired: 1 in, 3 out]
        n331 = local read "Numeric sort  folder names ?"() -> (w738:bool)
        n332 = call "list - get folder names.vi"("Numeric sort?"=w738, "folder path"=w740) -> ("Array"=w741:string[], "OK"=w742:bool)  [unwired: 8 in]
        n333 = case shown="False" w742 {
          selector: w742 -> [w743 w744]
          tunnel: w737 -> [_ w746]
          tunnel: w741 -> [_ w745]
          tunnel: [w743 w744] -> w739
          frame False {
          }
          frame True {
            n334 = property class="Ring (strict)"(reference=w746, "Strings []"=w745) -> ()  [unwired: 1 in, 2 out]
          }
        }
        n335 = local write "folder --OK"(w739) -> ()
      }
      event "sweep folder 1", "sweep folder 2": Value Change {
        n336 = event-data() -> ("CtlRef"=w758:refnum<vi>)  [unwired: 1 in]
        n337 = property class="Ring (strict)"(reference=w758) -> ("Label.Text"=w757:string, "Strings []"=w748:string[], "Value"=w747:u16)  [unwired: 1 in, 2 out]
        n338 = xnode "Match Regular Expression"("input string"=w757, "regular expression"=".*?(\\d+)") -> ("submatch 1"=w755:string)  [unwired: 4 in, 5 out]
        n339 = Index Array(array=w748, index=w747) -> (element=w753:string)
        n340 = Decimal String To Number(string=w755) -> (number=w754:i32)  [unwired: 2 in, 1 out]
        n341 = Build Path(base path=w752, name or relative path=w753) -> (appended path=w751:path)
        n342 = case shown="1, Default" w754 {
          tunnel: w751 -> [w760 w762]
          tunnel: ["update file path 1" ("event data") "update file path 2" ("event data")] -> w750
          frame 1, Default {
            n343 = local write "folder 1"(w760) -> ()
          }
          frame 2 {
            n344 = local write "folder 2"(w762) -> ()
          }
        }
        n345 = Generate User Event(user event=w749, event data cluster=w750) -> ()  [unwired: 2 in, 2 out]
      }
      event "Plot: frequency": Cursor Move {
        n346 = event-data() -> ("CursIdx"=w877:i32)  [unwired: 1 in, 3 out]
        n347 = call "cursor window logic V2.vi"("CursIdx"=w877, "cursor window action"=cursor_window_action."cursor moves", "cursor window in"=w876) -> ()  [unwired: 7 in, 2 out]
      }
      event "lockin (l)": Value Change {
        w881 = 2.0 ("Maximum")
        w880 = -2.0 ("Minimum")
        n348 = event-data() -> ()  [unwired: 1 in, 1 out]
        n349 = control-ref of="Plot: lockin"() -> (w879:refnum<vi>)
        n350 = property on="Property Node" class="XYGraph (strict)"(reference=w879, "XScale.Maximum"=w881, "XScale.Minimum"=w880, "YScale.Maximum"=w881, "YScale.Minimum"=w880) -> ()  [unwired: 1 in, 2 out]
        n351 = Generate User Event(user event=w882, event data cluster="poor man lockin" ("event data")) -> ()  [unwired: 2 in, 2 out]
      }
      event "period (min)": Value Change {
        n352 = event-data() -> ("NewVal"=w885:dbl)  [unwired: 1 in]
        n353 = local write "Lockin wave: Period (min)"(w885) -> ()
        n354 = Generate User Event(user event=w886, event data cluster="poor man lockin" ("event data")) -> ()  [unwired: 2 in, 2 out]
      }
      event "Plot: temp vs time": Cursor Release {
        n355 = event-data() -> ("CursIdx"=w889:i32)  [unwired: 1 in, 3 out]
        n356 = case shown="2..4" w889 {
          tunnel: w890 -> [_ _]
          tunnel: w888 -> [_ w891]
          frame 0, Default {
          }
          frame 2..4 {
            n357 = disable-structure shown="Disabled" {
              disable-tunnel: w891 -> [w893 _]
              frame Disabled {
                n358 = Generate User Event(user event=w893, event data cluster="update fit" ("event data")) -> ()  [unwired: 2 in, 2 out]
              }
              frame Enabled {
              }
            }
            n359 = Generate User Event(user event=w891, event data cluster="update slope" ("event data")) -> ()  [unwired: 2 in, 2 out]
          }
        }
      }
      event "fit dataset": Value Change {
        n360 = event-data() -> ("NewVal"=w898:enum16{"fit blue dataset", "fit red  dataset"})  [unwired: 1 in]
        n361 = case shown="\"fit blue dataset\", Default" w898 {
          tunnel: [u32 11589887 u32 16752849] -> w895
          frame "fit blue dataset", Default {
          }
          frame "fit red  dataset" {
          }
        }
        n362 = control-ref of="fit dataset"() -> (w897:refnum<vi>)
        n363 = property class="Enum (strict)"(reference=w897, "RingText.BGColor"=w895, "RingText.TextColor"=u32 460551) -> ()  [unwired: 1 in, 2 out]
      }
      event Value Change {
        n364 = event-data() -> ()  [unwired: 1 in, 1 out]
        n365 = Generate User Event(user event=w901, event data cluster="update fit" ("event data")) -> ()  [unwired: 2 in, 2 out]
      }
    }
    n366 = Wait (ms)(milliseconds to wait=u32 1) -> ()  [unwired: 1 out]
  }
  n367 = control-ref of="timer  \"update\""() -> (w43:refnum<vi>)
  n368 = call "slider timer .vi"("action"=countdown_control."start", "timer ref"=w43) -> ("timer out"=w42:refnum<vi>)  [unwired: 7 in, 2 out]
  n369 = while {
    shift-right: [w907] -> _
    shift-left: w42 -> [w908]
    tunnel: w41 -> [w904]
    stop <- FALSE stop-if-true
    n370 = case shown="\"timer ON\", Default" "Tab: timer" {
      tunnel: w908 -> [w912 w916]
      tunnel: [w911 w916] -> w907
      tunnel: w904 -> [w909 _]
      frame "timer ON", Default {
        n371 = call "slider timer .vi"("action"=countdown_control."check", "timer ref"=w912) -> ("tic"=w910:bool, "timer out"=w911:refnum<vi>)  [unwired: 7 in, 1 out]
        n372 = case shown="True" w910 {
          tunnel: w909 -> [_ w914]
          frame False {
          }
          frame True {
            n373 = Generate User Event(user event=w914, event data cluster="read file" ("event data")) -> ()  [unwired: 2 in, 2 out]
          }
        }
      }
      frame "timer OFF" {
      }
    }
    n374 = Wait (ms)(milliseconds to wait=u32 123) -> ()  [unwired: 1 out]
  }
